vi "AES Encrypt.vi"(0 "Password.In":string, 2 "BitKeyType(256)":u16(ring)=256 items=["AES bit key 128"=128, "AES bit key 192"=192, "AES bit key 256"=256], 7 "PlainText.In":string, 11 "error in":errorcluster, 13 "nonce":u32=123456789) -> (8 "CypheredText out":string, 15 "error out":errorcluster)   [LabVIEW 2020, in "Library Commun.lvlib"]
doc: "AES.Encrypt VI takes string (plain text) and encrypts it with Advanced Encryption Standart (AES) algorithm. \nAES.Encrypt.vi allows reentrant execution.\n-------------------------------------------------------------------------------------------\nThis VI belongs to Server Lab tools at Labicom.net (www.labicom.net) project of remote and virtual laboratories, written by (c) Igor Titov, 2011."
uses:
  Library Commun.lvlib
panel:
  in  "Product information, copyright notice, list of conditions and disclaimer":string="Please visit http://www.labicom.net to learn about remote and virtual laboratories. With it's services and tools you can create remote and/or virtual laboratory and even make money on it.\n \nCopyright (C) 2011 Igor Titov igor.ev.titov@gmail.com\n\nAll rights reserved.\n\nRedistribution and use without modification, are permitted provided that the following conditions are met:\n\n    * Redistributions of source code must retain the above copyright notice, this list of conditions and the following disclaimer.\n    * Redistributions of source code and in binary form may be freely used in all sorts of projects (including commercial ones). It is not obligatory to place copyright notice, this list of conditions and the following disclaimer in your product but you must mention the source (www.labicom.net, Igor Titov) on the web-site of the product.\n    * Neither the name of \"Labicom\", \"labicom.net\", \"Igor Titov\", nor the names of its contributors may be used to endorse or promote products derived from this software without specific prior written permission (except in situations mentioned in the terms and conditions of use of the \"Labicom\").\n\nTHIS SOFTWARE IS PROVIDED BY THE COPYRIGHT HOLDERS AND CONTRIBUTORS \"AS IS\" AND ANY EXPRESS OR IMPLIED WARRANTIES, INCLUDING, BUT NOT LIMITED TO, THE IMPLIED WARRANTIES OF MERCHANTABILITY AND FITNESS FOR A PARTICULAR PURPOSE ARE DISCLAIMED. IN NO EVENT SHALL THE COPYRIGHT OWNER OR CONTRIBUTORS BE LIABLE FOR ANY DIRECT, INDIRECT, INCIDENTAL, SPECIAL, EXEMPLARY, OR CONSEQUENTIAL DAMAGES (INCLUDING, BUT NOT LIMITED TO, PROCUREMENT OF SUBSTITUTE GOODS OR SERVICES; LOSS OF USE, DATA, OR PROFITS; OR BUSINESS INTERRUPTION) HOWEVER CAUSED AND ON ANY THEORY OF LIABILITY, \nWHETHER IN CONTRACT, STRICT LIABILITY, OR TORT (INCLUDING NEGLIGENCE OR OTHERWISE) ARISING IN ANY WAY OUT OF THE USE OF THIS SOFTWARE, EVEN IF ADVISED OF THE POSSIBILITY OF SUCH DAMAGE. "
  in  "Mix Bytes Phases":T1(ring)
  in  "Encryption Phases":T2(ring)
  out "cipherCharStr":string[](array[string])
  out "cipherChar":i32[](array[numeric])
  out "blockLength":i32
  out "cipherCntr":u16[](array[numeric])
  in  "0x100000000":u64=4294967296 format="%.0x"
  out "blockCount":i32
  in  "blockSize":i32=16
  in  "0xff":u16=255 format="%.0x"
  # "Real lab at YOUR home"
  # "Virtual & Remote Laboratories\nwww.labicom.net"
  # "Number of bits used in the key (256 by default).\nThe longer a key, the higher level of protection\nat expence of processor and RAM usage."
  # "Advanced Encryption Standart (AES)\nAES.Encrypt 1.0"
  # "Receives Password in String format (plain text)"
  # "Receives plain text needed to be encrypted"
  # "Encrypted text (with AES)"
  # "o?e?Ae§Oo??)y?B,\no?e?Ae§Oo??)y?B,UoV\"\nQoyµAv"
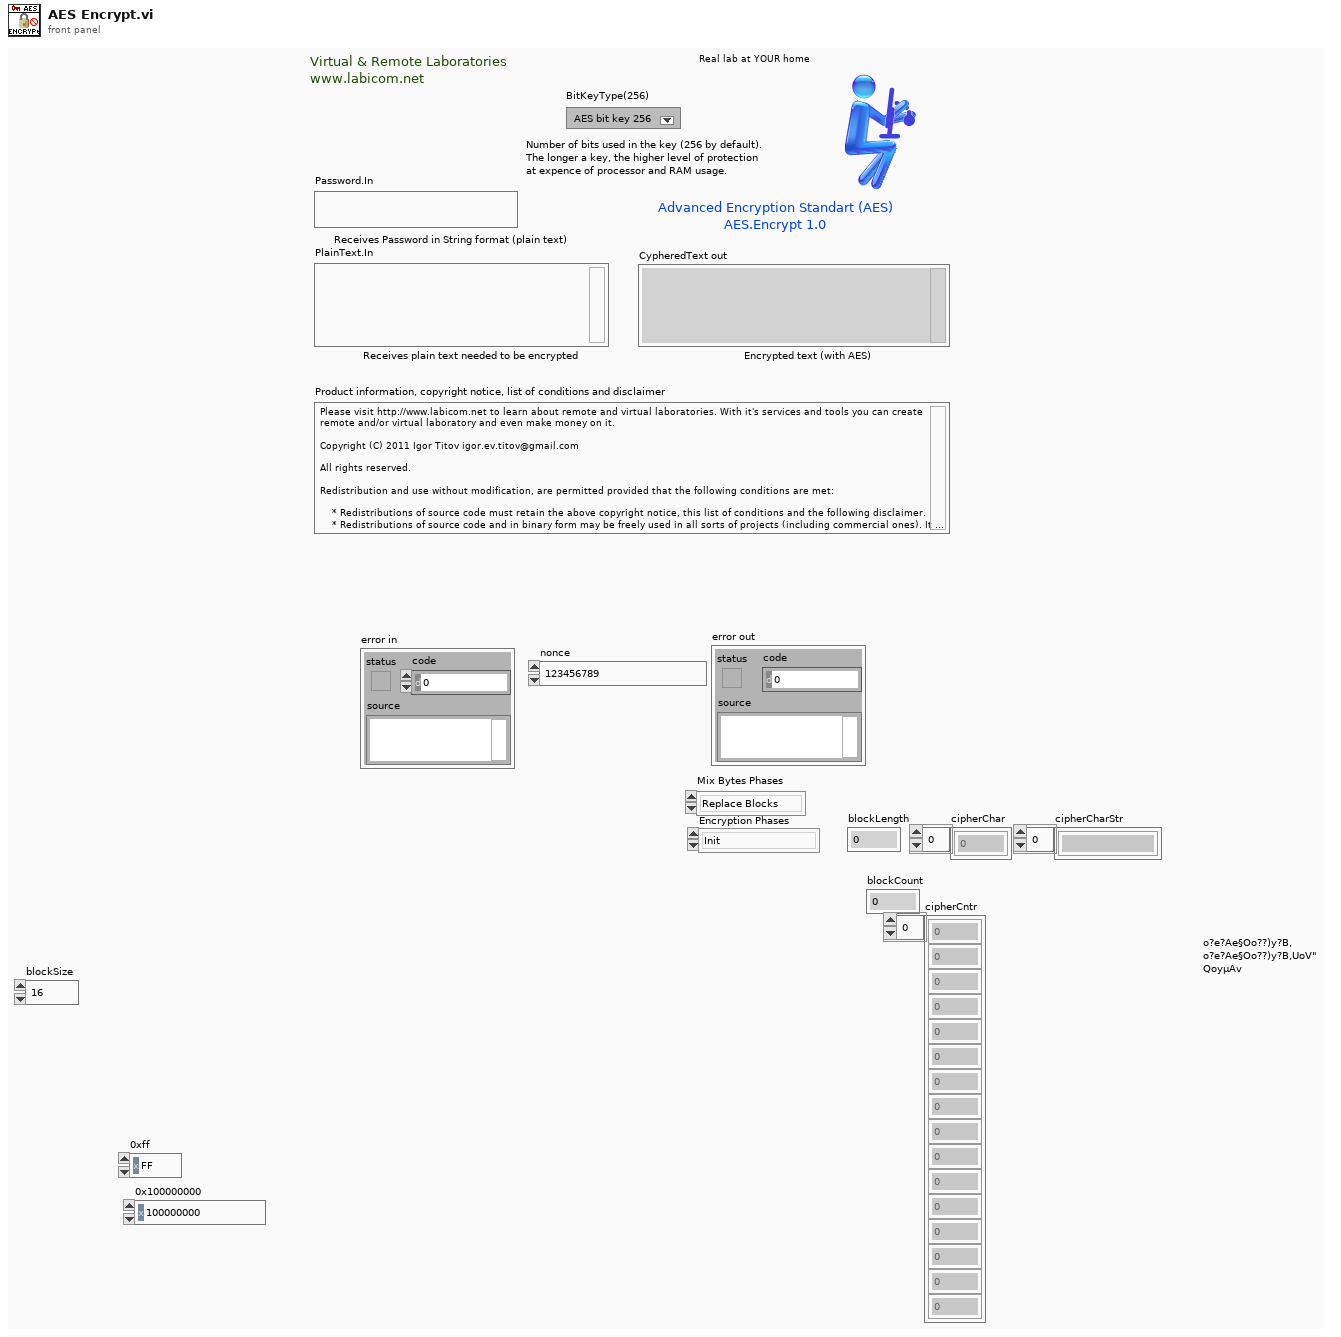
[diagram p1: front panel]
types:
  T1 = enum16{"Replace Blocks", "Cipher Blocks", "Replace ciphered", "Combine parts"}
  T2 = enum16{"Init", "Write pwBytes", "Create Key", "MixBlocks", "ToB64"}
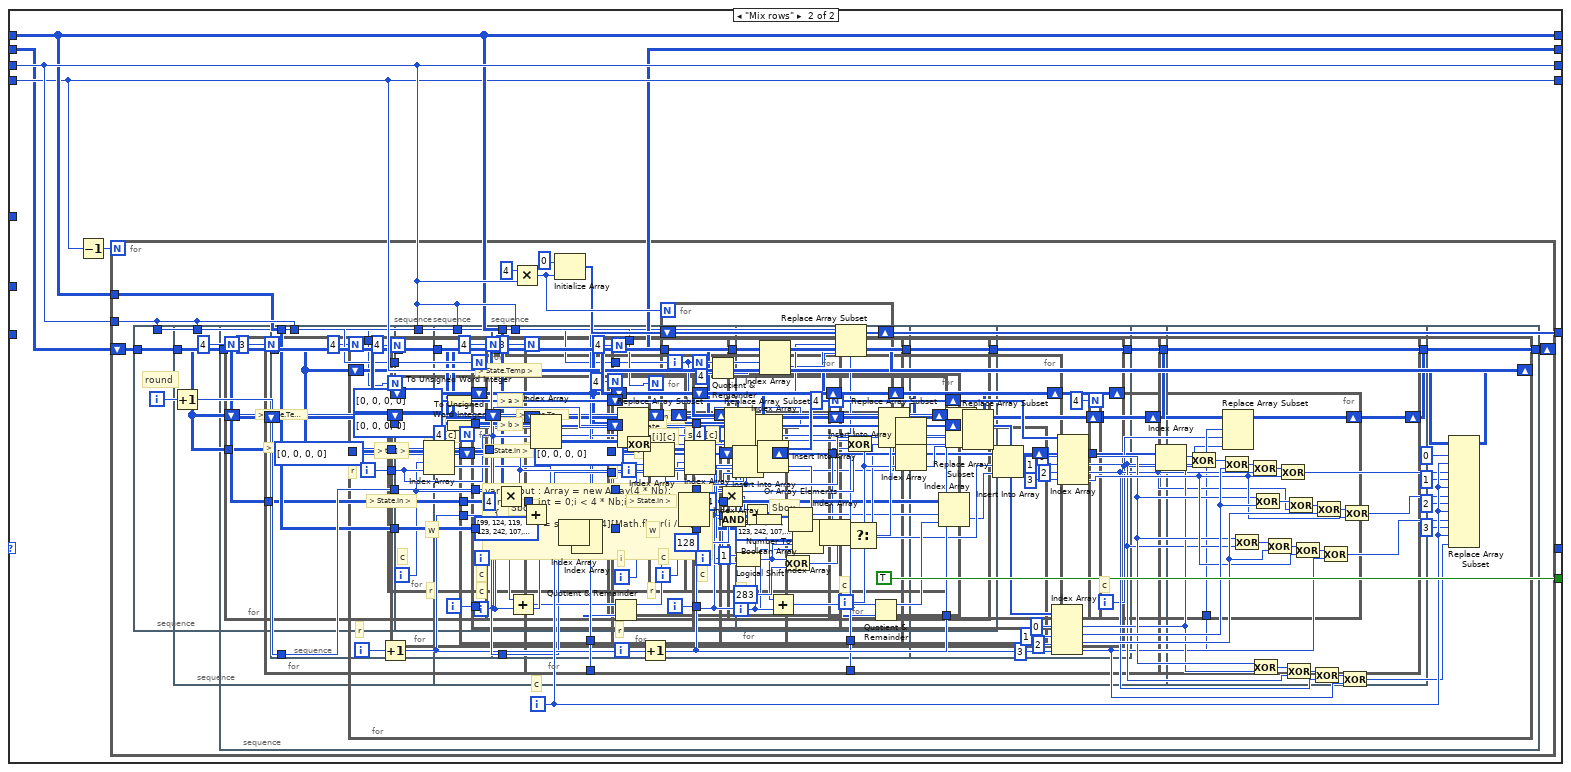
[diagram p4: hidden frame]
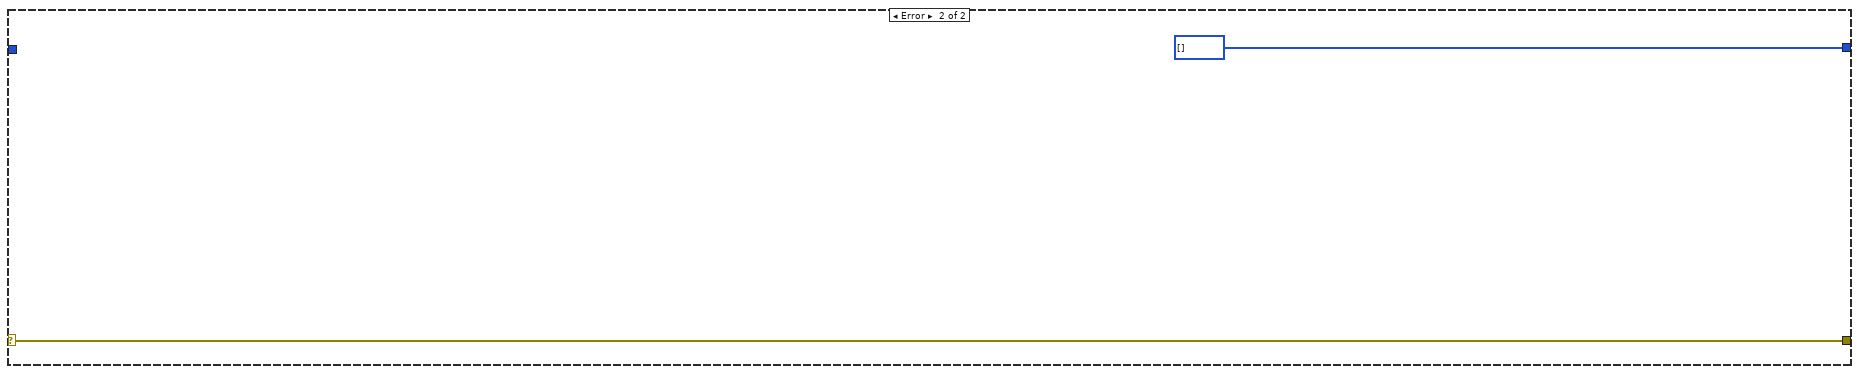
[diagram p5: hidden frame]
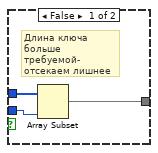
[diagram p6: hidden frame]
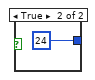
[diagram p7: hidden frame]
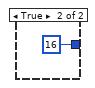
[diagram p8: hidden frame]
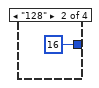
[diagram p9: hidden frame]
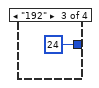
[diagram p10: hidden frame]
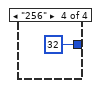
[diagram p11: hidden frame]
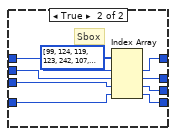
[diagram p12: hidden frame]
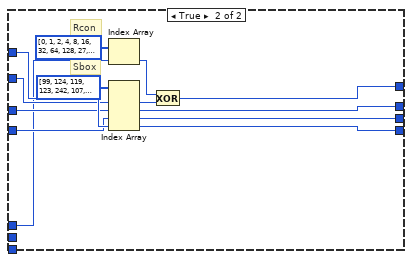
[diagram p13: hidden frame]
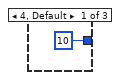
[diagram p14: hidden frame]
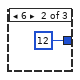
[diagram p15: hidden frame]
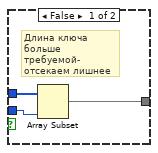
[diagram p16: hidden frame]
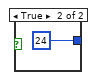
[diagram p17: hidden frame]
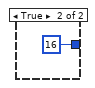
[diagram p18: hidden frame]
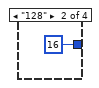
[diagram p19: hidden frame]
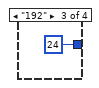
[diagram p20: hidden frame]
diagram:
  n1 = Quotient & Remainder(x="nonce", y=u32 1000) -> (x-y*floor(x/y)=w6:u32, floor(x/y)=w5:u32)
  n2 = case shown="Pas d'erreur" "error in" {
    selector: "error in" -> [w12 w1272]
    tunnel: [w20 w1272] -> w10
    tunnel: "Encryption Phases" -> [w19 _]
    tunnel: w6 -> [w18 _]
    tunnel: w5 -> [w17 _]
    tunnel: "PlainText.In" -> [w16 _]
    tunnel: "Password.In" -> [w15 _]
    tunnel: "BitKeyType(256)" -> [w14 _]
    tunnel: [w13 "" ("Base64 String")] -> w1
    frame No Error {
      n3 = Text to UTF-8(8:w12, 11:w16) -> (0:w20:errorcluster, 3:w21:string)  [unwired: 1 in]
      n4 = while {
        shift-right: [w33] -> _
        shift-left: w19 -> [w49]
        tunnel: w15 -> [w48]
        tunnel: w14 -> [w47]
        shift-right: [w45] -> _
        shift-left: _ -> [w41]
        shift-right: [w44] -> _
        shift-left: _ -> [w40]
        shift-right: [w43] -> _
        shift-left: _ -> [w42]
        shift-right: [w32] -> _
        shift-left: w21 -> [w46]
        shift-right: [w39] -> _
        shift-left: _ -> [w38]
        shift-right: [w37] -> _
        shift-left: _ -> [w36]
        shift-right: [w35] -> _
        shift-left: _ -> [w34]
        shift-right: [w31] -> _
        shift-left: _ -> [w30]
        shift-right: [w29] -> _
        shift-left: _ -> [w28]
        shift-right: [w27] -> _
        shift-left: _ -> [w26]
        tunnel: [w24] -> w13
        tunnel: w18 -> [w23]
        tunnel: w17 -> [w22]
        stop <- w25 stop-if-true
        # "> nonceSec >"
        # "> nonceMs >"
        # "> keySchedule >"
        # "> cipherTxt >"
        # "> ctrTxt >"
        # "> PasswordBytes >"
        # "> blockCount >"
        # "> blockSize >"
        # "> counterBlock >"
        # "> nBytes >"
        # "> PlainText >"
        # "> pwBytes >"
        n5 = case shown="\"Create Key\"" w49 {
          tunnel: w48 -> [w64 _ _ _ _]
          tunnel: w47 -> [w63 _ _ _ _]
          tunnel: w46 -> [w56 w76 w119 w745 w1217]
          tunnel: [w50 w77 w118 w746 w1218] -> w45
          tunnel: [w62 w75 w117 w744 w1216] -> w44
          tunnel: [w61 w84 w116 w743 w1215] -> w43
          tunnel: w42 -> [_ w85 w116 w743 w1215]
          tunnel: w41 -> [_ w77 w118 w746 w1218]
          tunnel: w40 -> [_ w75 w117 w744 w1216]
          tunnel: [w60 w82 w124 w748 w1220] -> w39
          tunnel: w38 -> [_ w83 w124 w748 w1220]
          tunnel: ["blockSize" w81 w120 w747 w1219] -> w37
          tunnel: w36 -> [_ w81 w120 w747 w1219]
          tunnel: [0 w79 w115 w742 w1214] -> w35
          tunnel: w34 -> [_ _ w115 w742 w1214]
          tunnel: [T2."Write pwBytes" ("Encryption Phases") T2."Create Key" ("Encryption Phases") T2."MixBlocks" ("Encryption Phases") T2."ToB64" ("Encryption Phases") T2."Init" ("Encryption Phases")] -> w33
          tunnel: [w56 w76 w119 w745 w1217] -> w32
          tunnel: [w55 w74 w123 w741 w1212] -> w31
          tunnel: w30 -> [_ w74 _ w741 w1212]
          tunnel: [w55 w73 "" w749 w1211] -> w29
          tunnel: w28 -> [_ w73 _ _ w1211]
          tunnel: [u16[] [] ("ExpandedKey") w72 w121 w740 w1213] -> w27
          tunnel: w26 -> [_ w72 _ w740 w1213]
          tunnel: [FALSE FALSE FALSE FALSE TRUE] -> w25
          tunnel: ["" ("Base64 String") _ _ _ w1221] -> w24
          tunnel: w23 -> [_ w71 _ _ _]
          tunnel: w22 -> [_ w70 _ _ _]
          frame "Init", Default {
            w55 = "" ("string")
            # "> counterBlock >"
            # "> pwBytes >"
            # "> nBytes >"
            n6 = Text to UTF-8(11:w64) -> (3:w68:string)  [unwired: 2 in, 1 out]
            n7 = String To Byte Array(string=w68) -> (unsigned byte array=w62:u8[])
            n8 = Divide(x=w63, y=u16 8) -> (x/y=w57:dbl)
            n9 = Initialize Array(u32 0 ("y"), "blockSize") -> (w60:u32[])
            n10 = Initialize Array(u32 0 ("element"), w57) -> (w61:u32[])
            n11 = To Long Integer(number=w57) -> (32bit integer=w50:i32)
          }
          frame "Write pwBytes" {
            # "> blockCount >"
            n12 = String Length(string=w76) -> (length=w87:i32)
            n13 = Divide(x=w87, y=w81) -> (x/y=w88:dbl)
            n14 = Round Toward +Infinity(x=w88) -> (ceil(x): smallest int >= x=w80:dbl)
            n15 = To Long Integer(number=w80) -> (32bit integer=w79:i32)
            "blockCount" <- w79
            n16 = for {
              N: w77 -> [_]
              tunnel: w75 -> [w104] mode=indexing
              shift-right: [w103] -> w84
              shift-left: w85 -> [w102]
              i -> [w106]
              n17 = Not A Number/Path/Refnum?(number/path/refnum=w104) -> (NaN/Path/Refnum?=w108:bool)
              n18 = Select(t=0 ("f"), s=w108, f=w104) -> (s? t:f=w107:i32)
              n19 = Replace Array Subset(array=w102, new element=w107, index=w106) -> (w103:u32[])
            }
            n20 = for {
              N: 4 -> [_]
              shift-right: [w93] -> w82
              shift-left: w83 -> [w92]
              tunnel: w71 -> [w90]
              tunnel: w70 -> [w89]
              i -> [w96]
              w91 = u16 255 ("0xff")
              n21 = Multiply(x=-8, y=w96) -> (x*y=w100:i32)
              n22 = Logical Shift(y=w100, x=w89) -> (x << y=w99:u32)
              n23 = And(x=w99, y=w91) -> (x .and. y?=w98:u32)
              n24 = And(x=w90, y=w91) -> (x .and. y?=w95:u32)
              n25 = Add(x=4, y=w96) -> (x+y=w94:i32)
              n26 = Replace Array Subset(array=w92, new element #1=w98, index #1=w96, new element #2=w95, index #2=w94) -> (w93:u32[])
            }
          }
          frame "Create Key" {
            # "> keySchedule >"
            # "> cipherTxt >"
            # "> ctrTxt >"
            # "> key >"
            n27 = stacked-sequence {
              tunnel: enum16{"128", "192", "256", "auto"}."auto" ("Mode (auto)") -> [w472]
              tunnel: w116 -> [w477]
              tunnel: [w478] -> w126
              frame #0 {
                n28 = Array Size(array=w477) -> (size(s)=w473:i32)
                n29 = case shown="\"auto\", Par défaut" w472 {
                  tunnel: w473 -> [w487 _ _ _]
                  tunnel: [w488 16 24 32] -> w475
                  frame "auto", Default {
                    n30 = Less Or Equal?(x=w487, y=16) -> (x <= y?=w489:bool)
                    n31 = case shown="Faux" w489 {
                      tunnel: [w491 16] -> w488
                      tunnel: w487 -> [w494 _]
                      frame False {
                        n32 = Less Or Equal?(x=w494, y=24) -> (x <= y?=w492:bool)
                        n33 = case shown="Faux" w492 {
                          tunnel: [32 ("y") 24 ("y")] -> w491
                          frame False {
                          }
                          frame True {
                          }
                        }
                      }
                      frame True {
                      }
                    }
                  }
                  frame "128" {
                  }
                  frame "192" {
                  }
                  frame "256" {
                  }
                }
                n34 = Less?(x=w473, y=w475) -> (x < y?=w474:bool)
                n35 = case shown="Vrai" w474 {
                  tunnel: w477 -> [w481 w482]
                  tunnel: w475 -> [w480 w486]
                  tunnel: [w479 w484] -> w476
                  frame False {
                    # "Длина ключа\nбольше требуемой-\nотсекаем лишнее"
                    n36 = Array Subset(array=w481, length=w480) -> (w479:u32[])  [unwired: 1 in]
                  }
                  frame True {
                    # "Длина ключа\nменьше требуемой-\nдополняем нулями"
                    n37 = Initialize Array(u32 0, w486) -> (w485:u32[])
                    n38 = Replace Array Subset(array=w485, new element=w482) -> (w484:u32[])  [unwired: 1 in]
                  }
                }
                n39 = Array Size(array=w476) -> (size(s)=w471:i32)
                n40 = Logical Shift(y=i8 -2, x=w471) -> (x << y=w464:i32)
                n41 = case shown="8" w464 {
                  tunnel: [10 12 14] -> w461
                  frame 4, Default {
                  }
                  frame 6 {
                  }
                  frame 8 {
                  }
                }
                n42 = Increment(x=w461) -> (x+1=w462:i32)
                n43 = Multiply(x=4, y=w462) -> (x*y=w468:i32)
                n44 = Logical Shift(y=i8 2, x=w468) -> (x << y=w467:i32)
                n45 = Initialize Array(u32 0 ("element"), w467) -> (w469:u32[])
                n46 = Replace Array Subset(array=w469, new element=w476) -> (w470:u32[])  [unwired: 1 in]
                n47 = while {
                  tunnel: w468 -> [w553]
                  tunnel: w464 -> [w533]
                  shift-right: [w510] -> w478
                  shift-left: w470 -> [w534]
                  tunnel: w475 -> [w532]
                  i -> [w554]
                  stop <- w552 continue-if-true
                  n48 = Add(x=w533, y=w554) -> (x+y=w536:i32)
                  n49 = Less?(x=w536, y=w553) -> (x < y?=w552:bool)
                  n50 = Quotient & Remainder(x=w536, y=w533) -> (x-y*floor(x/y)=w541:i32, floor(x/y)=w535:i32)
                  n51 = Logical Shift(y=i8 2, x=w536) -> (x << y=w505:i32)
                  n52 = Equal To 0?(x=w541) -> (x = 0?=w542:bool)
                  n53 = Subtract(x=w505, y=4) -> (x-y=w546:i32)
                  n54 = Subtract(x=w505, y=3) -> (x-y=w545:i32)
                  n55 = Subtract(x=w505, y=2) -> (x-y=w544:i32)
                  n56 = Subtract(x=w505, y=1) -> (x-y=w543:i32)
                  n57 = Index Array(array=w534, index #1=w546, index #2=w545, index #3=w544, index #4=w543) -> (element #1=w540:u32, element #2=w539:u32, element #3=w538:u32, element #4=w537:u32)
                  n58 = case shown="Faux" w542 {
                    tunnel: w533 -> [w569 _]
                    tunnel: w541 -> [w567 _]
                    tunnel: w540 -> [w562 w595]
                    tunnel: w539 -> [w561 w594]
                    tunnel: w538 -> [w560 w593]
                    tunnel: w537 -> [w559 w592]
                    tunnel: w535 -> [_ w591]
                    tunnel: [w558 w588] -> w514
                    tunnel: [w557 w587] -> w513
                    tunnel: [w556 w586] -> w512
                    tunnel: [w555 w585] -> w511
                    frame False {
                      n59 = Greater?(x=w569, y=6) -> (0:w565:bool)
                      n60 = Equal?(x=w567, y=4) -> (x = y?=w564:bool)
                      n61 = And(x=w565, y=w564) -> (x .and. y?=w563:bool)
                      n62 = case shown="Faux" w563 {
                        tunnel: w562 -> [w573 w582]
                        tunnel: w561 -> [w572 w581]
                        tunnel: w560 -> [w571 w580]
                        tunnel: w559 -> [w570 w579]
                        tunnel: [w573 w578] -> w558
                        tunnel: [w572 w577] -> w557
                        tunnel: [w571 w576] -> w556
                        tunnel: [w570 w575] -> w555
                        frame False {
                        }
                        frame True {
                          # "Sbox"
                          n63 = Index Array(array=u32[] [99, 124, 119, 123, 242, 107, 111, 197, 48, 1, 103, 43, 254, 215, 171, 118, 202, 130, 201, 125, 250, 89, 71, 240, 173, 212, 162, 175, 156, 164, 114, 192, 183, 253, 147, 38, 54, 63, 247, 204, 52, 165, 229, 241, 113, 216, 49, 21, 4, 199, 35, 195, 24, 150, 5, 154, 7, 18, 128, 226, 235, 39, 178, 117, 9, 131, 44, 26, 27, 110, 90, 160, 82, 59, 214, 179, 41, 227, 47, 132, 83, 209, 0, 237, 32, 252, 177, 91, 106, 203, 190, 57, 74, 76, 88, 207, 208, 239, 170, 251, 67, 77, 51, 133, 69, 249, 2, 127, 80, 60, 159, 168, 81, 163, 64, 143, 146, 157, 56, 245, 188, 182, 218, 33, 16, 255, 243, 210, 205, 12, 19, 236, 95, 151, 68, 23, 196, 167, 126, 61, 100, 93, 25, 115, 96, 129, 79, 220, 34, 42, 144, 136, 70, 238, 184, 20, 222, 94, 11, 219, 224, 50, 58, 10, 73, 6, 36, 92, 194, 211, 172, 98, 145, 149, 228, 121, 231, 200, 55, 109, 141, 213, 78, 169, 108, 86, 244, 234, 101, 122, 174, 8, 186, 120, 37, 46, 28, 166, 180, 198, 232, 221, 116, 31, 75, 189, 139, 138, 112, 62, 181, 102, 72, 3, 246, 14, 97, 53, 87, 185, 134, 193, 29, 158, 225, 248, 152, 17, 105, 217, 142, 148, 155, 30, 135, 233, 206, 85, 40, 223, 140, 161, 137, 13, 191, 230, 66, 104, 65, 153, 45, 15, 176, 84, 187, 22] ("Sbox"), index #1=w582, index #2=w581, index #3=w580, index #4=w579) -> (element #1=w578:u32, element #2=w577:u32, element #3=w576:u32, element #4=w575:u32)
                        }
                      }
                    }
                    frame True {
                      # "Sbox"
                      # "Rcon"
                      n64 = Index Array(array=u32[] [0, 1, 2, 4, 8, 16, 32, 64, 128, 27, 54] ("Rcon"), index=w591) -> (element=w590:u32)
                      n65 = Index Array(array=u32[] [99, 124, 119, 123, 242, 107, 111, 197, 48, 1, 103, 43, 254, 215, 171, 118, 202, 130, 201, 125, 250, 89, 71, 240, 173, 212, 162, 175, 156, 164, 114, 192, 183, 253, 147, 38, 54, 63, 247, 204, 52, 165, 229, 241, 113, 216, 49, 21, 4, 199, 35, 195, 24, 150, 5, 154, 7, 18, 128, 226, 235, 39, 178, 117, 9, 131, 44, 26, 27, 110, 90, 160, 82, 59, 214, 179, 41, 227, 47, 132, 83, 209, 0, 237, 32, 252, 177, 91, 106, 203, 190, 57, 74, 76, 88, 207, 208, 239, 170, 251, 67, 77, 51, 133, 69, 249, 2, 127, 80, 60, 159, 168, 81, 163, 64, 143, 146, 157, 56, 245, 188, 182, 218, 33, 16, 255, 243, 210, 205, 12, 19, 236, 95, 151, 68, 23, 196, 167, 126, 61, 100, 93, 25, 115, 96, 129, 79, 220, 34, 42, 144, 136, 70, 238, 184, 20, 222, 94, 11, 219, 224, 50, 58, 10, 73, 6, 36, 92, 194, 211, 172, 98, 145, 149, 228, 121, 231, 200, 55, 109, 141, 213, 78, 169, 108, 86, 244, 234, 101, 122, 174, 8, 186, 120, 37, 46, 28, 166, 180, 198, 232, 221, 116, 31, 75, 189, 139, 138, 112, 62, 181, 102, 72, 3, 246, 14, 97, 53, 87, 185, 134, 193, 29, 158, 225, 248, 152, 17, 105, 217, 142, 148, 155, 30, 135, 233, 206, 85, 40, 223, 140, 161, 137, 13, 191, 230, 66, 104, 65, 153, 45, 15, 176, 84, 187, 22] ("Sbox"), index #1=w594, index #2=w593, index #3=w592, index #4=w595) -> (element #1=w589:u32, element #2=w587:u32, element #3=w586:u32, element #4=w585:u32)
                      n66 = Exclusive Or(1:w589, 2:w590) -> (0:w588:u32)
                    }
                  }
                  n67 = Subtract(x=w505, y=w532) -> (x-y=w531:i32)
                  n68 = Add(x=w531, y=0) -> (x+y=w526:i32)
                  n69 = Add(x=w531, y=1) -> (x+y=w525:i32)
                  n70 = Add(x=w531, y=2) -> (x+y=w524:i32)
                  n71 = Add(x=w531, y=3) -> (x+y=w523:i32)
                  n72 = Index Array(array=w534, index #1=w526, index #2=w525, index #3=w524, index #4=w523) -> (element #1=w522:u32, element #2=w521:u32, element #3=w520:u32, element #4=w519:u32)
                  n73 = Exclusive Or(1:w514, 2:w522) -> (0:w518:u32)
                  n74 = Exclusive Or(1:w513, 2:w521) -> (0:w517:u32)
                  n75 = Exclusive Or(1:w512, 2:w520) -> (0:w516:u32)
                  n76 = Exclusive Or(1:w511, 2:w519) -> (0:w515:u32)
                  n77 = Add(x=w505, y=0) -> (x+y=w504:i32)
                  n78 = Add(x=w505, y=1) -> (x+y=w503:i32)
                  n79 = Add(x=w505, y=2) -> (x+y=w502:i32)
                  n80 = Add(x=w505, y=3) -> (x+y=w501:i32)
                  n81 = Replace Array Subset(array=w534, new element #1=w518, index #1=w504, new element #2=w517, index #2=w503, new element #3=w516, index #3=w502, new element #4=w515, index #4=w501) -> (w510:u32[])
                }
              }
            }
            n82 = Split 1D Array(array=w124, index=8) -> (first subarray=w135:u32[])  [unwired: 1 out]
            n83 = Subtract(x=w118, y=u8 16) -> (x-y=w131:i32)
            n84 = stacked-sequence {
              tunnel: w116 -> [w139]
              tunnel: [w140] -> w127
              tunnel: w126 -> [w138]
              tunnel: errorcluster {"status"=FALSE, "code"=0, "source"=""} ("error in") -> [w136]
              tunnel: [w137] -> _
              frame #0 {
                n85 = case shown="Pas d'erreur" w136 {
                  selector: w136 -> [_ w459]
                  tunnel: [_ w459] -> w137
                  tunnel: w138 -> [w145 _]
                  tunnel: w139 -> [w144 _]
                  tunnel: [w143 u16[] []] -> w140
                  tunnel: 4 ("Nb") -> [w142 _]
                  frame No Error {
                    n86 = while {
                      shift-right: [w149] -> _
                      shift-left: enum16{"Init", "Mix rows"}."Init" ("Cipher Phases") -> [w161]
                      tunnel: w145 -> [w160]
                      tunnel: w144 -> [w159]
                      shift-right: [w158] -> _
                      shift-left: _ -> [w157]
                      shift-right: [w156] -> _
                      shift-left: _ -> [w155]
                      shift-right: [w154] -> _
                      shift-left: _ -> [w153]
                      shift-right: [w152] -> _
                      shift-left: _ -> [w151]
                      tunnel: [w150] -> w143
                      tunnel: w142 -> [w147]
                      stop <- w148 stop-if-true
                      # "> Nr >"
                      # "> Nb >"
                      # "> State >"
                      # "> ExpandedKez(w)(2D) >"
                      n87 = case shown="\"Init\", Par défaut" w161 {
                        tunnel: w160 -> [w174 _]
                        tunnel: w159 -> [w172 _]
                        tunnel: [w169 w222] -> w158
                        tunnel: w157 -> [_ w222]
                        tunnel: [w168 w215] -> w156
                        tunnel: w155 -> [_ w216]
                        tunnel: [w162 w223] -> w154
                        tunnel: w153 -> [_ w223]
                        tunnel: [w166 w221] -> w152
                        tunnel: w151 -> [_ w221]
                        tunnel: [_ w218] -> w150
                        tunnel: [enum16{"Init", "Mix rows"}."Mix rows" ("Cipher Phases") _] -> w149
                        tunnel: [FALSE TRUE] -> w148
                        tunnel: w147 -> [w162 _]
                        frame "Init", Default {
                          # "> Nb >"
                          # "> ExpandedKey(w)(2D) >"
                          # "> Nr >"
                          n88 = Reshape Array(w174, 60 ("dimension size"), 4 ("dimension size")) -> (w169:u32[][])
                          n89 = for {
                            N: 16 -> [_]
                            tunnel: w172 -> [w209]
                            shift-right: [w207] -> w170
                            shift-left: u16[][] [[0, 0, 0, 0], [0, 0, 0, 0], [0, 0, 0, 0], [0, 0, 0, 0]] ("State.Out") -> [w208]
                            i -> [w214]
                            n90 = Quotient & Remainder(x=w214, y=4) -> (x-y*floor(x/y)=w211:i32, floor(x/y)=w210:i32)
                            n91 = Index Array(array=w209, index=w214) -> (element=w212:u32)
                            n92 = Replace Array Subset(array=w208, new element=w212, index (row)=w211, index (col)=w210) -> (w207:u16[][])
                          }
                          n93 = Array Size(array=w169) -> (size(s)=w175:i32[])
                          n94 = Index Array(array=w175, index=0) -> (element=w178:i32)
                          n95 = Divide(x=w178, y=w162) -> (x/y=w177:dbl)
                          n96 = Decrement(x=w177) -> (x-1=w167:dbl)
                          n97 = To Long Integer(number=w167) -> (32bit integer=w166:i32)
                          n98 = stacked-sequence {
                            tunnel: w169 -> [w181]
                            tunnel: w162 -> [w183]
                            tunnel: w170 -> [w185]
                            tunnel: [w186] -> w168
                            tunnel: 0 ("rnd (0)") -> [w184]
                            frame #0 {
                              n99 = for {
                                N: 4 -> [_]
                                tunnel: w185 -> [w192]
                                tunnel: w181 -> [w191]
                                tunnel: w183 -> [w190]
                                tunnel: w184 -> [w189]
                                shift-right: [w187] -> w186
                                shift-left: w185 -> [w188]
                                i -> [w193]
                                # "w"
                                # "state"
                                # "r"
                                n100 = for {
                                N: w190 -> [_]
                                tunnel: w193 -> [w198]
                                tunnel: w192 -> [w201]
                                tunnel: w191 -> [w206]
                                tunnel: w189 -> [w205]
                                shift-right: [w194] -> w187
                                shift-left: w188 -> [w195]
                                i -> [w197]
                                # "c"
                                n101 = Multiply(x=w205, y=4) -> (x*y=w203:i32)
                                n102 = Add(x=w203, y=w197) -> (x+y=w202:i32)
                                n103 = Index Array(array=w201, index (row)=w198, index (col)=w197) -> (element=w200:u16)
                                n104 = Index Array(array=w206, index (row)=w202, index (col)=w198) -> (element=w199:u32)
                                n105 = Exclusive Or(1:w199, 2:w200) -> (0:w196:u32)
                                n106 = Replace Array Subset(array=w195, new element=w196, index (row)=w198, index (col)=w197) -> (w194:u16[][])
                                }
                              }
                            }
                          }
                        }
                        frame "Mix rows" {
                          # "var output : Array = new Array(4 * Nb); \n\tfor (var i : int = 0;i < 4 * Nb;i++)\n   {\n    output[i] = state[i % 4][Math.floor(i / 4)];\n\t\t\t}"
                          n107 = Decrement(x=w221) -> (x-1=w229:i32)
                          n108 = for {
                            N: w229 -> [_]
                            shift-right: [w312] -> w224
                            shift-left: w216 -> [w313]
                            tunnel: w223 -> [w311]
                            tunnel: w222 -> [w310]
                            i -> [w315]
                            # "round"
                            n109 = stacked-sequence {
                              tunnel: w311 -> [w319]
                              tunnel: w313 -> [w321]
                              tunnel: [w322] -> w318
                              frame #0 {
                                n110 = for {
                                N: 4 -> [_]
                                tunnel: w321 -> [w326]
                                shift-right: [w323] -> w322
                                shift-left: w321 -> [w325]
                                tunnel: w319 -> [w324]
                                i -> [w327]
                                # "> State.In >"
                                # "> State.Temp >"
                                # "r"
                                n111 = for {
                                N: w324 -> [_]
                                tunnel: w326 -> [w335]
                                tunnel: w327 -> [w332]
                                shift-right: [w328] -> w323
                                shift-left: w325 -> [w329]
                                i -> [w331]
                                # "Sbox"
                                # "s[r][c]"
                                # "c"
                                n112 = Index Array(array=w335, index (row)=w331, index (col)=w332) -> (element=w334:u16)
                                n113 = Index Array(array=u16[] [99, 124, 119, 123, 242, 107, 111, 197, 48, 1, 103, 43, 254, 215, 171, 118, 202, 130, 201, 125, 250, 89, 71, 240, 173, 212, 162, 175, 156, 164, 114, 192, 183, 253, 147, 38, 54, 63, 247, 204, 52, 165, 229, 241, 113, 216, 49, 21, 4, 199, 35, 195, 24, 150, 5, 154, 7, 18, 128, 226, 235, 39, 178, 117, 9, 131, 44, 26, 27, 110, 90, 160, 82, 59, 214, 179, 41, 227, 47, 132, 83, 209, 0, 237, 32, 252, 177, 91, 106, 203, 190, 57, 74, 76, 88, 207, 208, 239, 170, 251, 67, 77, 51, 133, 69, 249, 2, 127, 80, 60, 159, 168, 81, 163, 64, 143, 146, 157, 56, 245, 188, 182, 218, 33, 16, 255, 243, 210, 205, 12, 19, 236, 95, 151, 68, 23, 196, 167, 126, 61, 100, 93, 25, 115, 96, 129, 79, 220, 34, 42, 144, 136, 70, 238, 184, 20, 222, 94, 11, 219, 224, 50, 58, 10, 73, 6, 36, 92, 194, 211, 172, 98, 145, 149, 228, 121, 231, 200, 55, 109, 141, 213, 78, 169, 108, 86, 244, 234, 101, 122, 174, 8, 186, 120, 37, 46, 28, 166, 180, 198, 232, 221, 116, 31, 75, 189, 139, 138, 112, 62, 181, 102, 72, 3, 246, 14, 97, 53, 87, 185, 134, 193, 29, 158, 225, 248, 152, 17, 105, 217, 142, 148, 155, 30, 135, 233, 206, 85, 40, 223, 140, 161, 137, 13, 191, 230, 66, 104, 65, 153, 45, 15, 176, 84, 187, 22] ("Sbox"), index=w334) -> (element=w333:u16)
                                n114 = Replace Array Subset(array=w329, new element=w333, index (row)=w331, index (col)=w332) -> (w328:u16[][])
                                }
                                }
                              }
                            }
                            n115 = Increment(x=w315) -> (x+1=w314:i32)
                            n116 = stacked-sequence {
                              tunnel: w311 -> [w336]
                              tunnel: w318 -> [w338]
                              tunnel: [w339] -> w317
                              frame #0 {
                                n117 = for {
                                N: 3 -> [_]
                                tunnel: w338 -> [w349]
                                shift-right: [w345] -> w339
                                shift-left: w338 -> [w346]
                                tunnel: w336 -> [w340]
                                i -> [w348]
                                # "> t[c] >"
                                # "> State.In >"
                                # "> State.Temp >"
                                # "r"
                                n118 = Increment(x=w348) -> (x+1=w347:i32)
                                n119 = for {
                                N: 4 -> [_]
                                tunnel: w349 -> [w364]
                                tunnel: w347 -> [w360]
                                shift-right: [w356] -> w343
                                shift-left: i32[] [0, 0, 0, 0] ("t[c]") -> [w357]
                                tunnel: w340 -> [w362]
                                i -> [w359]
                                # "c"
                                n120 = Add(x=w360, y=w359) -> (x+y=w363:i32)
                                n121 = Quotient & Remainder(x=w363, y=w362) -> (x-y*floor(x/y)=w361:i32)  [unwired: 1 out]
                                n122 = Index Array(array=w364, index (row)=w360, index (col)=w361) -> (element=w358:u16)
                                n123 = Insert Into Array(array=w357, index=w359, new element=w358) -> (w356:i32[])
                                }
                                n124 = for {
                                N: 4 -> [_]
                                tunnel: w347 -> [w355]
                                shift-right: [w351] -> w345
                                shift-left: w346 -> [w352]
                                tunnel: w343 -> [w350]
                                i -> [w354]
                                # "c"
                                n125 = Index Array(array=w350, index=w354) -> (element=w353:i32)
                                n126 = Replace Array Subset(array=w352, new element=w353, index (row)=w355, index (col)=w354) -> (w351:u16[][])
                                }
                                }
                              }
                            }
                            n127 = stacked-sequence {
                              tunnel: w317 -> [w366]
                              tunnel: [w367] -> w316
                              frame #0 {
                                n128 = for {
                                N: 4 -> [_]
                                shift-right: [w411] -> w367
                                shift-left: w366 -> [w412]
                                tunnel: w366 -> [w413]
                                i -> [w414]
                                # "> b >"
                                # "> a >"
                                # "> State.In >"
                                # "> State.Temp >"
                                # "c"
                                n129 = To Unsigned Word Integer(number=i32[] [0, 0, 0, 0] ("t[c]")) -> (unsigned 16bit integer=w408:u16[])
                                n130 = To Unsigned Word Integer(number=i32[] [0, 0, 0, 0] ("t[c]")) -> (unsigned 16bit integer=w407:u16[])
                                n131 = for {
                                N: 4 -> [_]
                                tunnel: w413 -> [w431]
                                tunnel: w414 -> [w430]
                                shift-right: [w417] -> w406
                                shift-left: w408 -> [w418]
                                shift-right: [w415] -> w405
                                shift-left: w407 -> [w416]
                                i -> [w429]
                                # "s[i][c]"
                                # "i"
                                n132 = Index Array(array=w431, index (row)=w429, index (col)=w430) -> (element=w423:u16)
                                n133 = And(x=w423, y=u16 128 ("0x80")) -> (x .and. y?=w426:u16)
                                n134 = Logical Shift(y=i8 1, x=w423) -> (x << y=w420:u16)
                                n135 = Number To Boolean Array(number=w426) -> (Boolean array=w425:bool[])
                                n136 = Insert Into Array(array=w418, index=w429, new element=w423) -> (w417:u16[])
                                n137 = Exclusive Or(1:u16 283 ("0x011b"), 2:w420) -> (0:w421:u16)
                                n138 = Or Array Elements(Boolean array=w425) -> (logical OR=w424:bool)
                                n139 = Select(t=w421, s=w424, f=w420) -> (s? t:f=w428:u16)
                                n140 = Insert Into Array(array=w416, index=w429, new element=w428) -> (w415:u16[])
                                }
                                n141 = Index Array(array=w405, index #1=0 ("index"), index #2=1 ("index"), index #3=2 ("index"), index #4=3 ("index")) -> (element #1=w376:u16, element #2=w388:u16, element #3=w383:u16, element #4=w373:u16)
                                n142 = Index Array(array=w406, index #1=0 ("index"), index #2=1 ("index"), index #3=2 ("index"), index #4=3 ("index")) -> (element #1=w377:u16, element #2=w375:u16, element #3=w374:u16, element #4=w382:u16)
                                n143 = Exclusive Or(1:w375, 2:w376) -> (0:w395:u16)
                                n144 = Exclusive Or(1:w388, 2:w395) -> (0:w394:u16)
                                n145 = Exclusive Or(1:w375, 2:w377) -> (0:w386:u16)
                                n146 = Exclusive Or(1:w374, 2:w394) -> (0:w393:u16)
                                n147 = Exclusive Or(1:w376, 2:w377) -> (0:w380:u16)
                                n148 = Exclusive Or(1:w388, 2:w377) -> (0:w391:u16)
                                n149 = Exclusive Or(1:w383, 2:w386) -> (0:w385:u16)
                                n150 = Exclusive Or(1:w382, 2:w393) -> (0:w392:u16)
                                n151 = Exclusive Or(1:w375, 2:w380) -> (0:w379:u16)
                                n152 = Exclusive Or(1:w374, 2:w391) -> (0:w390:u16)
                                n153 = Exclusive Or(1:w382, 2:w385) -> (0:w384:u16)
                                n154 = Exclusive Or(1:w374, 2:w379) -> (0:w378:u16)
                                n155 = Exclusive Or(1:w383, 2:w390) -> (0:w389:u16)
                                n156 = Exclusive Or(1:w373, 2:w384) -> (0:w381:u16)
                                n157 = Exclusive Or(1:w373, 2:w378) -> (0:w372:u16)
                                n158 = Exclusive Or(1:w382, 2:w389) -> (0:w387:u16)
                                n159 = Replace Array Subset(array=w412, new element #1=w392, index (row) #1=0 ("disabled index (col)"), index (col) #1=w414, new element #2=w387, index (row) #2=1 ("disabled index (col)"), index (col) #2=w414, new element #3=w381, index (row) #3=2 ("disabled index (col)"), index (col) #3=w414, new element #4=w372, index (row) #4=3 ("disabled index (col)"), index (col) #4=w414) -> (w411:u16[][])
                                }
                              }
                            }
                            n160 = stacked-sequence {
                              tunnel: w310 -> [w432]
                              tunnel: w311 -> [w434]
                              tunnel: w316 -> [w436]
                              tunnel: [w437] -> w312
                              tunnel: w314 -> [w435]
                              frame #0 {
                                n161 = for {
                                N: 4 -> [_]
                                tunnel: w436 -> [w443]
                                tunnel: w432 -> [w442]
                                tunnel: w434 -> [w441]
                                tunnel: w435 -> [w440]
                                shift-right: [w438] -> w437
                                shift-left: w436 -> [w439]
                                i -> [w444]
                                # "w"
                                # "state"
                                # "r"
                                n162 = for {
                                N: w441 -> [_]
                                tunnel: w444 -> [w449]
                                tunnel: w443 -> [w452]
                                tunnel: w442 -> [w457]
                                tunnel: w440 -> [w456]
                                shift-right: [w445] -> w438
                                shift-left: w439 -> [w446]
                                i -> [w448]
                                # "c"
                                n163 = Multiply(x=w456, y=4) -> (x*y=w454:i32)
                                n164 = Add(x=w454, y=w448) -> (x+y=w453:i32)
                                n165 = Index Array(array=w452, index (row)=w449, index (col)=w448) -> (element=w451:u16)
                                n166 = Index Array(array=w457, index (row)=w453, index (col)=w449) -> (element=w450:u32)
                                n167 = Exclusive Or(1:w450, 2:w451) -> (0:w447:u32)
                                n168 = Replace Array Subset(array=w446, new element=w447, index (row)=w449, index (col)=w448) -> (w445:u16[][])
                                }
                                }
                              }
                            }
                          }
                          n169 = stacked-sequence {
                            tunnel: w223 -> [w285]
                            tunnel: w224 -> [w287]
                            tunnel: [w288] -> w228
                            frame #0 {
                              n170 = for {
                                N: 4 -> [_]
                                tunnel: w287 -> [w292]
                                shift-right: [w289] -> w288
                                shift-left: w287 -> [w291]
                                tunnel: w285 -> [w290]
                                i -> [w293]
                                # "> State.In >"
                                # "> State.Temp >"
                                # "r"
                                n171 = for {
                                N: w290 -> [_]
                                tunnel: w292 -> [w301]
                                tunnel: w293 -> [w298]
                                shift-right: [w294] -> w289
                                shift-left: w291 -> [w295]
                                i -> [w297]
                                # "Sbox"
                                # "s[r][c]"
                                # "c"
                                n172 = Index Array(array=w301, index (row)=w297, index (col)=w298) -> (element=w300:u16)
                                n173 = Index Array(array=u16[] [99, 124, 119, 123, 242, 107, 111, 197, 48, 1, 103, 43, 254, 215, 171, 118, 202, 130, 201, 125, 250, 89, 71, 240, 173, 212, 162, 175, 156, 164, 114, 192, 183, 253, 147, 38, 54, 63, 247, 204, 52, 165, 229, 241, 113, 216, 49, 21, 4, 199, 35, 195, 24, 150, 5, 154, 7, 18, 128, 226, 235, 39, 178, 117, 9, 131, 44, 26, 27, 110, 90, 160, 82, 59, 214, 179, 41, 227, 47, 132, 83, 209, 0, 237, 32, 252, 177, 91, 106, 203, 190, 57, 74, 76, 88, 207, 208, 239, 170, 251, 67, 77, 51, 133, 69, 249, 2, 127, 80, 60, 159, 168, 81, 163, 64, 143, 146, 157, 56, 245, 188, 182, 218, 33, 16, 255, 243, 210, 205, 12, 19, 236, 95, 151, 68, 23, 196, 167, 126, 61, 100, 93, 25, 115, 96, 129, 79, 220, 34, 42, 144, 136, 70, 238, 184, 20, 222, 94, 11, 219, 224, 50, 58, 10, 73, 6, 36, 92, 194, 211, 172, 98, 145, 149, 228, 121, 231, 200, 55, 109, 141, 213, 78, 169, 108, 86, 244, 234, 101, 122, 174, 8, 186, 120, 37, 46, 28, 166, 180, 198, 232, 221, 116, 31, 75, 189, 139, 138, 112, 62, 181, 102, 72, 3, 246, 14, 97, 53, 87, 185, 134, 193, 29, 158, 225, 248, 152, 17, 105, 217, 142, 148, 155, 30, 135, 233, 206, 85, 40, 223, 140, 161, 137, 13, 191, 230, 66, 104, 65, 153, 45, 15, 176, 84, 187, 22] ("Sbox"), index=w300) -> (element=w299:u16)
                                n174 = Replace Array Subset(array=w295, new element=w299, index (row)=w297, index (col)=w298) -> (w294:u16[][])
                                }
                              }
                            }
                          }
                          n175 = stacked-sequence {
                            tunnel: w223 -> [w256]
                            tunnel: w228 -> [w258]
                            tunnel: [w259] -> w227
                            frame #0 {
                              n176 = for {
                                N: 3 -> [_]
                                tunnel: w258 -> [w269]
                                shift-right: [w265] -> w259
                                shift-left: w258 -> [w266]
                                tunnel: w256 -> [w260]
                                i -> [w268]
                                # "> t[c] >"
                                # "> State.In >"
                                # "> State.Temp >"
                                # "r"
                                n177 = Increment(x=w268) -> (x+1=w267:i32)
                                n178 = for {
                                N: 4 -> [_]
                                tunnel: w269 -> [w284]
                                tunnel: w267 -> [w280]
                                shift-right: [w276] -> w263
                                shift-left: i32[] [0, 0, 0, 0] ("t[c]") -> [w277]
                                tunnel: w260 -> [w282]
                                i -> [w279]
                                # "c"
                                n179 = Add(x=w280, y=w279) -> (x+y=w283:i32)
                                n180 = Quotient & Remainder(x=w283, y=w282) -> (x-y*floor(x/y)=w281:i32)  [unwired: 1 out]
                                n181 = Index Array(array=w284, index (row)=w280, index (col)=w281) -> (element=w278:u16)
                                n182 = Insert Into Array(array=w277, index=w279, new element=w278) -> (w276:i32[])
                                }
                                n183 = for {
                                N: 4 -> [_]
                                tunnel: w267 -> [w275]
                                shift-right: [w271] -> w265
                                shift-left: w266 -> [w272]
                                tunnel: w263 -> [w270]
                                i -> [w274]
                                # "c"
                                n184 = Index Array(array=w270, index=w274) -> (element=w273:i32)
                                n185 = Replace Array Subset(array=w272, new element=w273, index (row)=w275, index (col)=w274) -> (w271:u16[][])
                                }
                              }
                            }
                          }
                          n186 = stacked-sequence {
                            tunnel: w222 -> [w230]
                            tunnel: w223 -> [w232]
                            tunnel: w227 -> [w234]
                            tunnel: [w235] -> w215
                            tunnel: w221 -> [w233]
                            frame #0 {
                              n187 = for {
                                N: 4 -> [_]
                                tunnel: w234 -> [w241]
                                tunnel: w230 -> [w240]
                                tunnel: w232 -> [w239]
                                tunnel: w233 -> [w238]
                                shift-right: [w236] -> w235
                                shift-left: w234 -> [w237]
                                i -> [w242]
                                # "w"
                                # "state"
                                # "r"
                                n188 = for {
                                N: w239 -> [_]
                                tunnel: w242 -> [w247]
                                tunnel: w241 -> [w250]
                                tunnel: w240 -> [w255]
                                tunnel: w238 -> [w254]
                                shift-right: [w243] -> w236
                                shift-left: w237 -> [w244]
                                i -> [w246]
                                # "c"
                                n189 = Multiply(x=w254, y=4) -> (x*y=w252:i32)
                                n190 = Add(x=w252, y=w246) -> (x+y=w251:i32)
                                n191 = Index Array(array=w250, index (row)=w247, index (col)=w246) -> (element=w249:u16)
                                n192 = Index Array(array=w255, index (row)=w251, index (col)=w247) -> (element=w248:u32)
                                n193 = Exclusive Or(1:w248, 2:w249) -> (0:w245:u32)
                                n194 = Replace Array Subset(array=w244, new element=w245, index (row)=w247, index (col)=w246) -> (w243:u16[][])
                                }
                              }
                            }
                          }
                          n195 = Multiply(x=4, y=w223) -> (x*y=w220:i32)
                          n196 = Initialize Array(u16 0 ("x"), w220) -> (w219:u16[])
                          n197 = for {
                            N: w220 -> [_]
                            shift-right: [w302] -> w218
                            shift-left: w219 -> [w303]
                            tunnel: w215 -> [w304]
                            i -> [w306]
                            n198 = Quotient & Remainder(x=w306, y=4) -> (x-y*floor(x/y)=w308:i32, floor(x/y)=w307:i32)
                            n199 = Index Array(array=w304, index (row)=w308, index (col)=w307) -> (element=w305:u16)
                            n200 = Replace Array Subset(array=w303, new element=w305, index=w306) -> (w302:u16[])
                          }
                        }
                      }
                    }
                  }
                  frame Error {
                  }
                }
              }
            }
            n201 = Byte Array To String(unsigned byte array=w135) -> (string=w123:string)
            n202 = Byte Array To String(unsigned byte array=w127) -> (string=w128:string)
            n203 = String Subset(string=w128, offset (0)=0, length (rest)=w131) -> (substring=w132:string)
            n204 = Concatenate Strings(w128, w132) -> (w133:string)
            n205 = String To Byte Array(string=w133) -> (unsigned byte array=w114:u8[])
            n206 = To Unsigned Long Integer(number=w114) -> (unsigned 32bit integer=w113:u32[])
            n207 = stacked-sequence {
              tunnel: enum16{"128", "192", "256", "auto"}."auto" ("Mode (auto)") -> [w611]
              tunnel: w113 -> [w616]
              tunnel: [w617] -> w121
              frame #0 {
                n208 = Array Size(array=w616) -> (size(s)=w612:i32)
                n209 = case shown="\"auto\", Par défaut" w611 {
                  tunnel: w612 -> [w626 _ _ _]
                  tunnel: [w627 16 24 32] -> w614
                  frame "auto", Default {
                    n210 = Less Or Equal?(x=w626, y=16) -> (x <= y?=w628:bool)
                    n211 = case shown="Faux" w628 {
                      tunnel: [w630 16] -> w627
                      tunnel: w626 -> [w633 _]
                      frame False {
                        n212 = Less Or Equal?(x=w633, y=24) -> (x <= y?=w631:bool)
                        n213 = case shown="Faux" w631 {
                          tunnel: [32 ("y") 24 ("y")] -> w630
                          frame False {
                          }
                          frame True {
                          }
                        }
                      }
                      frame True {
                      }
                    }
                  }
                  frame "128" {
                  }
                  frame "192" {
                  }
                  frame "256" {
                  }
                }
                n214 = Less?(x=w612, y=w614) -> (x < y?=w613:bool)
                n215 = case shown="Vrai" w613 {
                  tunnel: w616 -> [w620 w621]
                  tunnel: w614 -> [w619 w625]
                  tunnel: [w618 w623] -> w615
                  frame False {
                    # "Длина ключа\nбольше требуемой-\nотсекаем лишнее"
                    n216 = Array Subset(array=w620, length=w619) -> (w618:u32[])  [unwired: 1 in]
                  }
                  frame True {
                    # "Длина ключа\nменьше требуемой-\nдополняем нулями"
                    n217 = Initialize Array(u32 0, w625) -> (w624:u32[])
                    n218 = Replace Array Subset(array=w624, new element=w621) -> (w623:u32[])  [unwired: 1 in]
                  }
                }
                n219 = Array Size(array=w615) -> (size(s)=w610:i32)
                n220 = Logical Shift(y=i8 -2, x=w610) -> (x << y=w603:i32)
                n221 = case shown="8" w603 {
                  tunnel: [10 12 14] -> w600
                  frame 4, Default {
                  }
                  frame 6 {
                  }
                  frame 8 {
                  }
                }
                n222 = Increment(x=w600) -> (x+1=w601:i32)
                n223 = Multiply(x=4, y=w601) -> (x*y=w607:i32)
                n224 = Logical Shift(y=i8 2, x=w607) -> (x << y=w606:i32)
                n225 = Initialize Array(u32 0 ("element"), w606) -> (w608:u32[])
                n226 = Replace Array Subset(array=w608, new element=w615) -> (w609:u32[])  [unwired: 1 in]
                n227 = while {
                  tunnel: w607 -> [w692]
                  tunnel: w603 -> [w672]
                  shift-right: [w649] -> w617
                  shift-left: w609 -> [w673]
                  tunnel: w614 -> [w671]
                  i -> [w693]
                  stop <- w691 continue-if-true
                  n228 = Add(x=w672, y=w693) -> (x+y=w675:i32)
                  n229 = Less?(x=w675, y=w692) -> (x < y?=w691:bool)
                  n230 = Quotient & Remainder(x=w675, y=w672) -> (x-y*floor(x/y)=w680:i32, floor(x/y)=w674:i32)
                  n231 = Logical Shift(y=i8 2, x=w675) -> (x << y=w644:i32)
                  n232 = Equal To 0?(x=w680) -> (x = 0?=w681:bool)
                  n233 = Subtract(x=w644, y=4) -> (x-y=w685:i32)
                  n234 = Subtract(x=w644, y=3) -> (x-y=w684:i32)
                  n235 = Subtract(x=w644, y=2) -> (x-y=w683:i32)
                  n236 = Subtract(x=w644, y=1) -> (x-y=w682:i32)
                  n237 = Index Array(array=w673, index #1=w685, index #2=w684, index #3=w683, index #4=w682) -> (element #1=w679:u32, element #2=w678:u32, element #3=w677:u32, element #4=w676:u32)
                  n238 = case shown="Faux" w681 {
                    tunnel: w672 -> [w708 _]
                    tunnel: w680 -> [w706 _]
                    tunnel: w679 -> [w701 w734]
                    tunnel: w678 -> [w700 w733]
                    tunnel: w677 -> [w699 w732]
                    tunnel: w676 -> [w698 w731]
                    tunnel: w674 -> [_ w730]
                    tunnel: [w697 w727] -> w653
                    tunnel: [w696 w726] -> w652
                    tunnel: [w695 w725] -> w651
                    tunnel: [w694 w724] -> w650
                    frame False {
                      n239 = Greater?(x=w708, y=6) -> (0:w704:bool)
                      n240 = Equal?(x=w706, y=4) -> (x = y?=w703:bool)
                      n241 = And(x=w704, y=w703) -> (x .and. y?=w702:bool)
                      n242 = case shown="Faux" w702 {
                        tunnel: w701 -> [w712 w721]
                        tunnel: w700 -> [w711 w720]
                        tunnel: w699 -> [w710 w719]
                        tunnel: w698 -> [w709 w718]
                        tunnel: [w712 w717] -> w697
                        tunnel: [w711 w716] -> w696
                        tunnel: [w710 w715] -> w695
                        tunnel: [w709 w714] -> w694
                        frame False {
                        }
                        frame True {
                          # "Sbox"
                          n243 = Index Array(array=u32[] [99, 124, 119, 123, 242, 107, 111, 197, 48, 1, 103, 43, 254, 215, 171, 118, 202, 130, 201, 125, 250, 89, 71, 240, 173, 212, 162, 175, 156, 164, 114, 192, 183, 253, 147, 38, 54, 63, 247, 204, 52, 165, 229, 241, 113, 216, 49, 21, 4, 199, 35, 195, 24, 150, 5, 154, 7, 18, 128, 226, 235, 39, 178, 117, 9, 131, 44, 26, 27, 110, 90, 160, 82, 59, 214, 179, 41, 227, 47, 132, 83, 209, 0, 237, 32, 252, 177, 91, 106, 203, 190, 57, 74, 76, 88, 207, 208, 239, 170, 251, 67, 77, 51, 133, 69, 249, 2, 127, 80, 60, 159, 168, 81, 163, 64, 143, 146, 157, 56, 245, 188, 182, 218, 33, 16, 255, 243, 210, 205, 12, 19, 236, 95, 151, 68, 23, 196, 167, 126, 61, 100, 93, 25, 115, 96, 129, 79, 220, 34, 42, 144, 136, 70, 238, 184, 20, 222, 94, 11, 219, 224, 50, 58, 10, 73, 6, 36, 92, 194, 211, 172, 98, 145, 149, 228, 121, 231, 200, 55, 109, 141, 213, 78, 169, 108, 86, 244, 234, 101, 122, 174, 8, 186, 120, 37, 46, 28, 166, 180, 198, 232, 221, 116, 31, 75, 189, 139, 138, 112, 62, 181, 102, 72, 3, 246, 14, 97, 53, 87, 185, 134, 193, 29, 158, 225, 248, 152, 17, 105, 217, 142, 148, 155, 30, 135, 233, 206, 85, 40, 223, 140, 161, 137, 13, 191, 230, 66, 104, 65, 153, 45, 15, 176, 84, 187, 22] ("Sbox"), index #1=w721, index #2=w720, index #3=w719, index #4=w718) -> (element #1=w717:u32, element #2=w716:u32, element #3=w715:u32, element #4=w714:u32)
                        }
                      }
                    }
                    frame True {
                      # "Sbox"
                      # "Rcon"
                      n244 = Index Array(array=u32[] [0, 1, 2, 4, 8, 16, 32, 64, 128, 27, 54] ("Rcon"), index=w730) -> (element=w729:u32)
                      n245 = Index Array(array=u32[] [99, 124, 119, 123, 242, 107, 111, 197, 48, 1, 103, 43, 254, 215, 171, 118, 202, 130, 201, 125, 250, 89, 71, 240, 173, 212, 162, 175, 156, 164, 114, 192, 183, 253, 147, 38, 54, 63, 247, 204, 52, 165, 229, 241, 113, 216, 49, 21, 4, 199, 35, 195, 24, 150, 5, 154, 7, 18, 128, 226, 235, 39, 178, 117, 9, 131, 44, 26, 27, 110, 90, 160, 82, 59, 214, 179, 41, 227, 47, 132, 83, 209, 0, 237, 32, 252, 177, 91, 106, 203, 190, 57, 74, 76, 88, 207, 208, 239, 170, 251, 67, 77, 51, 133, 69, 249, 2, 127, 80, 60, 159, 168, 81, 163, 64, 143, 146, 157, 56, 245, 188, 182, 218, 33, 16, 255, 243, 210, 205, 12, 19, 236, 95, 151, 68, 23, 196, 167, 126, 61, 100, 93, 25, 115, 96, 129, 79, 220, 34, 42, 144, 136, 70, 238, 184, 20, 222, 94, 11, 219, 224, 50, 58, 10, 73, 6, 36, 92, 194, 211, 172, 98, 145, 149, 228, 121, 231, 200, 55, 109, 141, 213, 78, 169, 108, 86, 244, 234, 101, 122, 174, 8, 186, 120, 37, 46, 28, 166, 180, 198, 232, 221, 116, 31, 75, 189, 139, 138, 112, 62, 181, 102, 72, 3, 246, 14, 97, 53, 87, 185, 134, 193, 29, 158, 225, 248, 152, 17, 105, 217, 142, 148, 155, 30, 135, 233, 206, 85, 40, 223, 140, 161, 137, 13, 191, 230, 66, 104, 65, 153, 45, 15, 176, 84, 187, 22] ("Sbox"), index #1=w733, index #2=w732, index #3=w731, index #4=w734) -> (element #1=w728:u32, element #2=w726:u32, element #3=w725:u32, element #4=w724:u32)
                      n246 = Exclusive Or(1:w728, 2:w729) -> (0:w727:u32)
                    }
                  }
                  n247 = Subtract(x=w644, y=w671) -> (x-y=w670:i32)
                  n248 = Add(x=w670, y=0) -> (x+y=w665:i32)
                  n249 = Add(x=w670, y=1) -> (x+y=w664:i32)
                  n250 = Add(x=w670, y=2) -> (x+y=w663:i32)
                  n251 = Add(x=w670, y=3) -> (x+y=w662:i32)
                  n252 = Index Array(array=w673, index #1=w665, index #2=w664, index #3=w663, index #4=w662) -> (element #1=w661:u32, element #2=w660:u32, element #3=w659:u32, element #4=w658:u32)
                  n253 = Exclusive Or(1:w653, 2:w661) -> (0:w657:u32)
                  n254 = Exclusive Or(1:w652, 2:w660) -> (0:w656:u32)
                  n255 = Exclusive Or(1:w651, 2:w659) -> (0:w655:u32)
                  n256 = Exclusive Or(1:w650, 2:w658) -> (0:w654:u32)
                  n257 = Add(x=w644, y=0) -> (x+y=w643:i32)
                  n258 = Add(x=w644, y=1) -> (x+y=w642:i32)
                  n259 = Add(x=w644, y=2) -> (x+y=w641:i32)
                  n260 = Add(x=w644, y=3) -> (x+y=w640:i32)
                  n261 = Replace Array Subset(array=w673, new element #1=w657, index #1=w643, new element #2=w656, index #2=w642, new element #3=w655, index #3=w641, new element #4=w654, index #4=w640) -> (w649:u32[])
                }
              }
            }
          }
          frame "MixBlocks" {
            n262 = for {
              N: w742 -> [w765]
              shift-right: [w767] -> _
              shift-left: w748 -> [w768]
              shift-right: [w751] -> _
              shift-left: w740 -> [w766]
              shift-right: [w756] -> _
              shift-left: w747 -> [w764]
              tunnel: w745 -> [w763]
              shift-right: [w762] -> _
              shift-left: _ -> [w761]
              shift-right: [w760] -> _
              shift-left: _ -> [w759]
              shift-right: [w758] -> _
              shift-left: _ -> [w757]
              shift-right: [w755] -> _
              shift-left: _ -> [w754]
              shift-right: [w753] -> w749
              shift-left: "" -> [w752]
              i -> [w769]
              # "> cipherTxt >"
              # "> cipherCntr >"
              # "> blockLength >"
              # "> cipherChar >"
              # "> cipherCharStr >"
              # "> PlainText >"
              # "> blockSize >"
              # "> keySchedule >"
              # "> counterBlock >"
              # "b"
              n263 = while {
                shift-right: [w791] -> _
                shift-left: "Mix Bytes Phases" -> [w792]
                tunnel: w769 -> [w789]
                shift-right: [w787] -> w767
                shift-left: w768 -> [w788]
                shift-right: [w784] -> w751
                shift-left: w766 -> [w786]
                tunnel: w765 -> [w785]
                shift-right: [w771] -> w756
                shift-left: w764 -> [w783]
                tunnel: w763 -> [w782]
                shift-right: [w781] -> w762
                shift-left: w761 -> [w772]
                shift-right: [w780] -> w760
                shift-left: w759 -> [w777]
                shift-right: [w779] -> w758
                shift-left: w757 -> [w778]
                shift-right: [w776] -> w755
                shift-left: w754 -> [w775]
                shift-right: [w774] -> w753
                shift-left: w752 -> [w773]
                stop <- w790 stop-if-true
                n264 = case shown="\"Cipher Blocks\"" w792 {
                  tunnel: [T1."Cipher Blocks" ("Mix Bytes Phases") T1."Replace ciphered" ("Mix Bytes Phases") T1."Combine parts" ("Mix Bytes Phases") T1."Replace Blocks" ("Mix Bytes Phases")] -> w791
                  tunnel: [FALSE FALSE FALSE TRUE] -> w790
                  tunnel: w789 -> [w802 w835 w1181 _]
                  tunnel: w788 -> [w801 w828 w1172 w1201]
                  tunnel: [w800 w828 w1172 w1201] -> w787
                  tunnel: w786 -> [w799 w827 w1171 w1200]
                  tunnel: w785 -> [_ w834 _ _]
                  tunnel: [w799 w827 w1171 w1200] -> w784
                  tunnel: w783 -> [w795 w826 w1173 w1199]
                  tunnel: w782 -> [_ w833 w1178 _]
                  tunnel: [string[] [] w832 w1176 w1204] -> w781
                  tunnel: [i32[] [] w831 w1177 w1203] -> w780
                  tunnel: [0 ("blockSize") w830 w1174 w1198] -> w779
                  tunnel: w778 -> [_ _ w1180 w1198]
                  tunnel: w777 -> [_ _ w1179 w1203]
                  tunnel: [u16[] [] ("Cypher.Output") w829 w1175 w1202] -> w776
                  tunnel: w775 -> [_ _ w1175 w1202]
                  tunnel: [w793 w825 w1170 w1206] -> w774
                  tunnel: w773 -> [w793 w825 w1170 w1205]
                  tunnel: w772 -> [_ _ w1176 w1204]
                  tunnel: [w795 w826 w1173 w1199] -> w771
                  frame "Replace Blocks", Default {
                    n265 = for {
                      N: 4 -> [_]
                      tunnel: w802 -> [w820]
                      tunnel: w802 -> [w813]
                      shift-right: [w806] -> w800
                      shift-left: w801 -> [w807]
                      i -> [w819]
                      # "c"
                      n266 = Divide(x=w813, y="0x100000000") -> (x/y=w811:dbl)
                      n267 = Multiply(x=-8, y=w819) -> (x*y=w812:i32)
                      n268 = Logical Shift(y=w812, x=w820) -> (x << y=w822:i32)
                      n269 = And(x=w822, y=u16 255 ("0xff")) -> (x .and. y?=w817:i32)
                      n270 = Subtract(x=15, y=w819) -> (x-y=w816:i32)
                      n271 = Logical Shift(y=w812, x=w811) -> (x << y=w810:u32)
                      n272 = Subtract(x=w816, y=4) -> (x-y=w814:i32)
                      n273 = Replace Array Subset(array=w807, new element #1=w817, index #1=w816, new element #2=w810, index #2=w814) -> (w806:u32[])
                    }
                  }
                  frame "Cipher Blocks" {
                    n274 = Decrement(x=w834) -> (x-1=w836:i32)
                    n275 = Greater?(x=w836, y=w835) -> (0:w837:bool)
                    n276 = String Length(string=w833) -> (length=w839:i32)
                    n277 = Decrement(x=w839) -> (x-1=w838:i32)
                    n278 = stacked-sequence {
                      tunnel: w828 -> [w848]
                      tunnel: [w849] -> w829
                      tunnel: w827 -> [w847]
                      tunnel: errorcluster {"status"=FALSE, "code"=0, "source"=""} ("error in") -> [w845]
                      tunnel: [w846] -> _
                      frame #0 {
                        n279 = case shown="Pas d'erreur" w845 {
                          selector: w845 -> [_ w1168]
                          tunnel: [_ w1168] -> w846
                          tunnel: w847 -> [w854 _]
                          tunnel: w848 -> [w853 _]
                          tunnel: [w852 u16[] []] -> w849
                          tunnel: 4 ("Nb") -> [w851 _]
                          frame No Error {
                            n280 = while {
                              shift-right: [w858] -> _
                              shift-left: enum16{"Init", "Mix rows"}."Init" ("Cipher Phases") -> [w870]
                              tunnel: w854 -> [w869]
                              tunnel: w853 -> [w868]
                              shift-right: [w867] -> _
                              shift-left: _ -> [w866]
                              shift-right: [w865] -> _
                              shift-left: _ -> [w864]
                              shift-right: [w863] -> _
                              shift-left: _ -> [w862]
                              shift-right: [w861] -> _
                              shift-left: _ -> [w860]
                              tunnel: [w859] -> w852
                              tunnel: w851 -> [w856]
                              stop <- w857 stop-if-true
                              # "> Nr >"
                              # "> Nb >"
                              # "> State >"
                              # "> ExpandedKez(w)(2D) >"
                              n281 = case shown="\"Init\", Par défaut" w870 {
                                tunnel: w869 -> [w883 _]
                                tunnel: w868 -> [w881 _]
                                tunnel: [w878 w931] -> w867
                                tunnel: w866 -> [_ w931]
                                tunnel: [w877 w924] -> w865
                                tunnel: w864 -> [_ w925]
                                tunnel: [w871 w932] -> w863
                                tunnel: w862 -> [_ w932]
                                tunnel: [w875 w930] -> w861
                                tunnel: w860 -> [_ w930]
                                tunnel: [_ w927] -> w859
                                tunnel: [enum16{"Init", "Mix rows"}."Mix rows" ("Cipher Phases") _] -> w858
                                tunnel: [FALSE TRUE] -> w857
                                tunnel: w856 -> [w871 _]
                                frame "Init", Default {
                                # "> Nb >"
                                # "> ExpandedKey(w)(2D) >"
                                # "> Nr >"
                                n282 = Reshape Array(w883, 60 ("dimension size"), 4 ("dimension size")) -> (w878:u32[][])
                                n283 = for {
                                N: 16 -> [_]
                                tunnel: w881 -> [w918]
                                shift-right: [w916] -> w879
                                shift-left: u16[][] [[0, 0, 0, 0], [0, 0, 0, 0], [0, 0, 0, 0], [0, 0, 0, 0]] ("State.Out") -> [w917]
                                i -> [w923]
                                n284 = Quotient & Remainder(x=w923, y=4) -> (x-y*floor(x/y)=w920:i32, floor(x/y)=w919:i32)
                                n285 = Index Array(array=w918, index=w923) -> (element=w921:u32)
                                n286 = Replace Array Subset(array=w917, new element=w921, index (row)=w920, index (col)=w919) -> (w916:u16[][])
                                }
                                n287 = Array Size(array=w878) -> (size(s)=w884:i32[])
                                n288 = Index Array(array=w884, index=0) -> (element=w887:i32)
                                n289 = Divide(x=w887, y=w871) -> (x/y=w886:dbl)
                                n290 = Decrement(x=w886) -> (x-1=w876:dbl)
                                n291 = To Long Integer(number=w876) -> (32bit integer=w875:i32)
                                n292 = stacked-sequence {
                                tunnel: w878 -> [w890]
                                tunnel: w871 -> [w892]
                                tunnel: w879 -> [w894]
                                tunnel: [w895] -> w877
                                tunnel: 0 ("rnd (0)") -> [w893]
                                frame #0 {
                                n293 = for {
                                N: 4 -> [_]
                                tunnel: w894 -> [w901]
                                tunnel: w890 -> [w900]
                                tunnel: w892 -> [w899]
                                tunnel: w893 -> [w898]
                                shift-right: [w896] -> w895
                                shift-left: w894 -> [w897]
                                i -> [w902]
                                # "w"
                                # "state"
                                # "r"
                                n294 = for {
                                N: w899 -> [_]
                                tunnel: w902 -> [w907]
                                tunnel: w901 -> [w910]
                                tunnel: w900 -> [w915]
                                tunnel: w898 -> [w914]
                                shift-right: [w903] -> w896
                                shift-left: w897 -> [w904]
                                i -> [w906]
                                # "c"
                                n295 = Multiply(x=w914, y=4) -> (x*y=w912:i32)
                                n296 = Add(x=w912, y=w906) -> (x+y=w911:i32)
                                n297 = Index Array(array=w910, index (row)=w907, index (col)=w906) -> (element=w909:u16)
                                n298 = Index Array(array=w915, index (row)=w911, index (col)=w907) -> (element=w908:u32)
                                n299 = Exclusive Or(1:w908, 2:w909) -> (0:w905:u32)
                                n300 = Replace Array Subset(array=w904, new element=w905, index (row)=w907, index (col)=w906) -> (w903:u16[][])
                                }
                                }
                                }
                                }
                                }
                                frame "Mix rows" {
                                # "var output : Array = new Array(4 * Nb); \n\tfor (var i : int = 0;i < 4 * Nb;i++)\n   {\n    output[i] = state[i % 4][Math.floor(i / 4)];\n\t\t\t}"
                                n301 = Decrement(x=w930) -> (x-1=w938:i32)
                                n302 = for {
                                N: w938 -> [_]
                                shift-right: [w1021] -> w933
                                shift-left: w925 -> [w1022]
                                tunnel: w932 -> [w1020]
                                tunnel: w931 -> [w1019]
                                i -> [w1024]
                                # "round"
                                n303 = stacked-sequence {
                                tunnel: w1020 -> [w1028]
                                tunnel: w1022 -> [w1030]
                                tunnel: [w1031] -> w1027
                                frame #0 {
                                n304 = for {
                                N: 4 -> [_]
                                tunnel: w1030 -> [w1035]
                                shift-right: [w1032] -> w1031
                                shift-left: w1030 -> [w1034]
                                tunnel: w1028 -> [w1033]
                                i -> [w1036]
                                # "> State.In >"
                                # "> State.Temp >"
                                # "r"
                                n305 = for {
                                N: w1033 -> [_]
                                tunnel: w1035 -> [w1044]
                                tunnel: w1036 -> [w1041]
                                shift-right: [w1037] -> w1032
                                shift-left: w1034 -> [w1038]
                                i -> [w1040]
                                # "Sbox"
                                # "s[r][c]"
                                # "c"
                                n306 = Index Array(array=w1044, index (row)=w1040, index (col)=w1041) -> (element=w1043:u16)
                                n307 = Index Array(array=u16[] [99, 124, 119, 123, 242, 107, 111, 197, 48, 1, 103, 43, 254, 215, 171, 118, 202, 130, 201, 125, 250, 89, 71, 240, 173, 212, 162, 175, 156, 164, 114, 192, 183, 253, 147, 38, 54, 63, 247, 204, 52, 165, 229, 241, 113, 216, 49, 21, 4, 199, 35, 195, 24, 150, 5, 154, 7, 18, 128, 226, 235, 39, 178, 117, 9, 131, 44, 26, 27, 110, 90, 160, 82, 59, 214, 179, 41, 227, 47, 132, 83, 209, 0, 237, 32, 252, 177, 91, 106, 203, 190, 57, 74, 76, 88, 207, 208, 239, 170, 251, 67, 77, 51, 133, 69, 249, 2, 127, 80, 60, 159, 168, 81, 163, 64, 143, 146, 157, 56, 245, 188, 182, 218, 33, 16, 255, 243, 210, 205, 12, 19, 236, 95, 151, 68, 23, 196, 167, 126, 61, 100, 93, 25, 115, 96, 129, 79, 220, 34, 42, 144, 136, 70, 238, 184, 20, 222, 94, 11, 219, 224, 50, 58, 10, 73, 6, 36, 92, 194, 211, 172, 98, 145, 149, 228, 121, 231, 200, 55, 109, 141, 213, 78, 169, 108, 86, 244, 234, 101, 122, 174, 8, 186, 120, 37, 46, 28, 166, 180, 198, 232, 221, 116, 31, 75, 189, 139, 138, 112, 62, 181, 102, 72, 3, 246, 14, 97, 53, 87, 185, 134, 193, 29, 158, 225, 248, 152, 17, 105, 217, 142, 148, 155, 30, 135, 233, 206, 85, 40, 223, 140, 161, 137, 13, 191, 230, 66, 104, 65, 153, 45, 15, 176, 84, 187, 22] ("Sbox"), index=w1043) -> (element=w1042:u16)
                                n308 = Replace Array Subset(array=w1038, new element=w1042, index (row)=w1040, index (col)=w1041) -> (w1037:u16[][])
                                }
                                }
                                }
                                }
                                n309 = Increment(x=w1024) -> (x+1=w1023:i32)
                                n310 = stacked-sequence {
                                tunnel: w1020 -> [w1045]
                                tunnel: w1027 -> [w1047]
                                tunnel: [w1048] -> w1026
                                frame #0 {
                                n311 = for {
                                N: 3 -> [_]
                                tunnel: w1047 -> [w1058]
                                shift-right: [w1054] -> w1048
                                shift-left: w1047 -> [w1055]
                                tunnel: w1045 -> [w1049]
                                i -> [w1057]
                                # "> t[c] >"
                                # "> State.In >"
                                # "> State.Temp >"
                                # "r"
                                n312 = Increment(x=w1057) -> (x+1=w1056:i32)
                                n313 = for {
                                N: 4 -> [_]
                                tunnel: w1058 -> [w1073]
                                tunnel: w1056 -> [w1069]
                                shift-right: [w1065] -> w1052
                                shift-left: i32[] [0, 0, 0, 0] ("t[c]") -> [w1066]
                                tunnel: w1049 -> [w1071]
                                i -> [w1068]
                                # "c"
                                n314 = Add(x=w1069, y=w1068) -> (x+y=w1072:i32)
                                n315 = Quotient & Remainder(x=w1072, y=w1071) -> (x-y*floor(x/y)=w1070:i32)  [unwired: 1 out]
                                n316 = Index Array(array=w1073, index (row)=w1069, index (col)=w1070) -> (element=w1067:u16)
                                n317 = Insert Into Array(array=w1066, index=w1068, new element=w1067) -> (w1065:i32[])
                                }
                                n318 = for {
                                N: 4 -> [_]
                                tunnel: w1056 -> [w1064]
                                shift-right: [w1060] -> w1054
                                shift-left: w1055 -> [w1061]
                                tunnel: w1052 -> [w1059]
                                i -> [w1063]
                                # "c"
                                n319 = Index Array(array=w1059, index=w1063) -> (element=w1062:i32)
                                n320 = Replace Array Subset(array=w1061, new element=w1062, index (row)=w1064, index (col)=w1063) -> (w1060:u16[][])
                                }
                                }
                                }
                                }
                                n321 = stacked-sequence {
                                tunnel: w1026 -> [w1075]
                                tunnel: [w1076] -> w1025
                                frame #0 {
                                n322 = for {
                                N: 4 -> [_]
                                shift-right: [w1120] -> w1076
                                shift-left: w1075 -> [w1121]
                                tunnel: w1075 -> [w1122]
                                i -> [w1123]
                                # "> b >"
                                # "> a >"
                                # "> State.In >"
                                # "> State.Temp >"
                                # "c"
                                n323 = To Unsigned Word Integer(number=i32[] [0, 0, 0, 0] ("t[c]")) -> (unsigned 16bit integer=w1117:u16[])
                                n324 = To Unsigned Word Integer(number=i32[] [0, 0, 0, 0] ("t[c]")) -> (unsigned 16bit integer=w1116:u16[])
                                n325 = for {
                                N: 4 -> [_]
                                tunnel: w1122 -> [w1140]
                                tunnel: w1123 -> [w1139]
                                shift-right: [w1126] -> w1115
                                shift-left: w1117 -> [w1127]
                                shift-right: [w1124] -> w1114
                                shift-left: w1116 -> [w1125]
                                i -> [w1138]
                                # "s[i][c]"
                                # "i"
                                n326 = Index Array(array=w1140, index (row)=w1138, index (col)=w1139) -> (element=w1132:u16)
                                n327 = And(x=w1132, y=u16 128 ("0x80")) -> (x .and. y?=w1135:u16)
                                n328 = Logical Shift(y=i8 1, x=w1132) -> (x << y=w1129:u16)
                                n329 = Number To Boolean Array(number=w1135) -> (Boolean array=w1134:bool[])
                                n330 = Insert Into Array(array=w1127, index=w1138, new element=w1132) -> (w1126:u16[])
                                n331 = Exclusive Or(1:u16 283 ("0x011b"), 2:w1129) -> (0:w1130:u16)
                                n332 = Or Array Elements(Boolean array=w1134) -> (logical OR=w1133:bool)
                                n333 = Select(t=w1130, s=w1133, f=w1129) -> (s? t:f=w1137:u16)
                                n334 = Insert Into Array(array=w1125, index=w1138, new element=w1137) -> (w1124:u16[])
                                }
                                n335 = Index Array(array=w1114, index #1=0 ("index"), index #2=1 ("index"), index #3=2 ("index"), index #4=3 ("index")) -> (element #1=w1085:u16, element #2=w1097:u16, element #3=w1092:u16, element #4=w1082:u16)
                                n336 = Index Array(array=w1115, index #1=0 ("index"), index #2=1 ("index"), index #3=2 ("index"), index #4=3 ("index")) -> (element #1=w1086:u16, element #2=w1084:u16, element #3=w1083:u16, element #4=w1091:u16)
                                n337 = Exclusive Or(1:w1084, 2:w1085) -> (0:w1104:u16)
                                n338 = Exclusive Or(1:w1097, 2:w1104) -> (0:w1103:u16)
                                n339 = Exclusive Or(1:w1084, 2:w1086) -> (0:w1095:u16)
                                n340 = Exclusive Or(1:w1083, 2:w1103) -> (0:w1102:u16)
                                n341 = Exclusive Or(1:w1085, 2:w1086) -> (0:w1089:u16)
                                n342 = Exclusive Or(1:w1097, 2:w1086) -> (0:w1100:u16)
                                n343 = Exclusive Or(1:w1092, 2:w1095) -> (0:w1094:u16)
                                n344 = Exclusive Or(1:w1091, 2:w1102) -> (0:w1101:u16)
                                n345 = Exclusive Or(1:w1084, 2:w1089) -> (0:w1088:u16)
                                n346 = Exclusive Or(1:w1083, 2:w1100) -> (0:w1099:u16)
                                n347 = Exclusive Or(1:w1091, 2:w1094) -> (0:w1093:u16)
                                n348 = Exclusive Or(1:w1083, 2:w1088) -> (0:w1087:u16)
                                n349 = Exclusive Or(1:w1092, 2:w1099) -> (0:w1098:u16)
                                n350 = Exclusive Or(1:w1082, 2:w1093) -> (0:w1090:u16)
                                n351 = Exclusive Or(1:w1082, 2:w1087) -> (0:w1081:u16)
                                n352 = Exclusive Or(1:w1091, 2:w1098) -> (0:w1096:u16)
                                n353 = Replace Array Subset(array=w1121, new element #1=w1101, index (row) #1=0 ("disabled index (col)"), index (col) #1=w1123, new element #2=w1096, index (row) #2=1 ("disabled index (col)"), index (col) #2=w1123, new element #3=w1090, index (row) #3=2 ("disabled index (col)"), index (col) #3=w1123, new element #4=w1081, index (row) #4=3 ("disabled index (col)"), index (col) #4=w1123) -> (w1120:u16[][])
                                }
                                }
                                }
                                n354 = stacked-sequence {
                                tunnel: w1019 -> [w1141]
                                tunnel: w1020 -> [w1143]
                                tunnel: w1025 -> [w1145]
                                tunnel: [w1146] -> w1021
                                tunnel: w1023 -> [w1144]
                                frame #0 {
                                n355 = for {
                                N: 4 -> [_]
                                tunnel: w1145 -> [w1152]
                                tunnel: w1141 -> [w1151]
                                tunnel: w1143 -> [w1150]
                                tunnel: w1144 -> [w1149]
                                shift-right: [w1147] -> w1146
                                shift-left: w1145 -> [w1148]
                                i -> [w1153]
                                # "w"
                                # "state"
                                # "r"
                                n356 = for {
                                N: w1150 -> [_]
                                tunnel: w1153 -> [w1158]
                                tunnel: w1152 -> [w1161]
                                tunnel: w1151 -> [w1166]
                                tunnel: w1149 -> [w1165]
                                shift-right: [w1154] -> w1147
                                shift-left: w1148 -> [w1155]
                                i -> [w1157]
                                # "c"
                                n357 = Multiply(x=w1165, y=4) -> (x*y=w1163:i32)
                                n358 = Add(x=w1163, y=w1157) -> (x+y=w1162:i32)
                                n359 = Index Array(array=w1161, index (row)=w1158, index (col)=w1157) -> (element=w1160:u16)
                                n360 = Index Array(array=w1166, index (row)=w1162, index (col)=w1158) -> (element=w1159:u32)
                                n361 = Exclusive Or(1:w1159, 2:w1160) -> (0:w1156:u32)
                                n362 = Replace Array Subset(array=w1155, new element=w1156, index (row)=w1158, index (col)=w1157) -> (w1154:u16[][])
                                }
                                }
                                }
                                }
                                }
                                n363 = stacked-sequence {
                                tunnel: w932 -> [w994]
                                tunnel: w933 -> [w996]
                                tunnel: [w997] -> w937
                                frame #0 {
                                n364 = for {
                                N: 4 -> [_]
                                tunnel: w996 -> [w1001]
                                shift-right: [w998] -> w997
                                shift-left: w996 -> [w1000]
                                tunnel: w994 -> [w999]
                                i -> [w1002]
                                # "> State.In >"
                                # "> State.Temp >"
                                # "r"
                                n365 = for {
                                N: w999 -> [_]
                                tunnel: w1001 -> [w1010]
                                tunnel: w1002 -> [w1007]
                                shift-right: [w1003] -> w998
                                shift-left: w1000 -> [w1004]
                                i -> [w1006]
                                # "Sbox"
                                # "s[r][c]"
                                # "c"
                                n366 = Index Array(array=w1010, index (row)=w1006, index (col)=w1007) -> (element=w1009:u16)
                                n367 = Index Array(array=u16[] [99, 124, 119, 123, 242, 107, 111, 197, 48, 1, 103, 43, 254, 215, 171, 118, 202, 130, 201, 125, 250, 89, 71, 240, 173, 212, 162, 175, 156, 164, 114, 192, 183, 253, 147, 38, 54, 63, 247, 204, 52, 165, 229, 241, 113, 216, 49, 21, 4, 199, 35, 195, 24, 150, 5, 154, 7, 18, 128, 226, 235, 39, 178, 117, 9, 131, 44, 26, 27, 110, 90, 160, 82, 59, 214, 179, 41, 227, 47, 132, 83, 209, 0, 237, 32, 252, 177, 91, 106, 203, 190, 57, 74, 76, 88, 207, 208, 239, 170, 251, 67, 77, 51, 133, 69, 249, 2, 127, 80, 60, 159, 168, 81, 163, 64, 143, 146, 157, 56, 245, 188, 182, 218, 33, 16, 255, 243, 210, 205, 12, 19, 236, 95, 151, 68, 23, 196, 167, 126, 61, 100, 93, 25, 115, 96, 129, 79, 220, 34, 42, 144, 136, 70, 238, 184, 20, 222, 94, 11, 219, 224, 50, 58, 10, 73, 6, 36, 92, 194, 211, 172, 98, 145, 149, 228, 121, 231, 200, 55, 109, 141, 213, 78, 169, 108, 86, 244, 234, 101, 122, 174, 8, 186, 120, 37, 46, 28, 166, 180, 198, 232, 221, 116, 31, 75, 189, 139, 138, 112, 62, 181, 102, 72, 3, 246, 14, 97, 53, 87, 185, 134, 193, 29, 158, 225, 248, 152, 17, 105, 217, 142, 148, 155, 30, 135, 233, 206, 85, 40, 223, 140, 161, 137, 13, 191, 230, 66, 104, 65, 153, 45, 15, 176, 84, 187, 22] ("Sbox"), index=w1009) -> (element=w1008:u16)
                                n368 = Replace Array Subset(array=w1004, new element=w1008, index (row)=w1006, index (col)=w1007) -> (w1003:u16[][])
                                }
                                }
                                }
                                }
                                n369 = stacked-sequence {
                                tunnel: w932 -> [w965]
                                tunnel: w937 -> [w967]
                                tunnel: [w968] -> w936
                                frame #0 {
                                n370 = for {
                                N: 3 -> [_]
                                tunnel: w967 -> [w978]
                                shift-right: [w974] -> w968
                                shift-left: w967 -> [w975]
                                tunnel: w965 -> [w969]
                                i -> [w977]
                                # "> t[c] >"
                                # "> State.In >"
                                # "> State.Temp >"
                                # "r"
                                n371 = Increment(x=w977) -> (x+1=w976:i32)
                                n372 = for {
                                N: 4 -> [_]
                                tunnel: w978 -> [w993]
                                tunnel: w976 -> [w989]
                                shift-right: [w985] -> w972
                                shift-left: i32[] [0, 0, 0, 0] ("t[c]") -> [w986]
                                tunnel: w969 -> [w991]
                                i -> [w988]
                                # "c"
                                n373 = Add(x=w989, y=w988) -> (x+y=w992:i32)
                                n374 = Quotient & Remainder(x=w992, y=w991) -> (x-y*floor(x/y)=w990:i32)  [unwired: 1 out]
                                n375 = Index Array(array=w993, index (row)=w989, index (col)=w990) -> (element=w987:u16)
                                n376 = Insert Into Array(array=w986, index=w988, new element=w987) -> (w985:i32[])
                                }
                                n377 = for {
                                N: 4 -> [_]
                                tunnel: w976 -> [w984]
                                shift-right: [w980] -> w974
                                shift-left: w975 -> [w981]
                                tunnel: w972 -> [w979]
                                i -> [w983]
                                # "c"
                                n378 = Index Array(array=w979, index=w983) -> (element=w982:i32)
                                n379 = Replace Array Subset(array=w981, new element=w982, index (row)=w984, index (col)=w983) -> (w980:u16[][])
                                }
                                }
                                }
                                }
                                n380 = stacked-sequence {
                                tunnel: w931 -> [w939]
                                tunnel: w932 -> [w941]
                                tunnel: w936 -> [w943]
                                tunnel: [w944] -> w924
                                tunnel: w930 -> [w942]
                                frame #0 {
                                n381 = for {
                                N: 4 -> [_]
                                tunnel: w943 -> [w950]
                                tunnel: w939 -> [w949]
                                tunnel: w941 -> [w948]
                                tunnel: w942 -> [w947]
                                shift-right: [w945] -> w944
                                shift-left: w943 -> [w946]
                                i -> [w951]
                                # "w"
                                # "state"
                                # "r"
                                n382 = for {
                                N: w948 -> [_]
                                tunnel: w951 -> [w956]
                                tunnel: w950 -> [w959]
                                tunnel: w949 -> [w964]
                                tunnel: w947 -> [w963]
                                shift-right: [w952] -> w945
                                shift-left: w946 -> [w953]
                                i -> [w955]
                                # "c"
                                n383 = Multiply(x=w963, y=4) -> (x*y=w961:i32)
                                n384 = Add(x=w961, y=w955) -> (x+y=w960:i32)
                                n385 = Index Array(array=w959, index (row)=w956, index (col)=w955) -> (element=w958:u16)
                                n386 = Index Array(array=w964, index (row)=w960, index (col)=w956) -> (element=w957:u32)
                                n387 = Exclusive Or(1:w957, 2:w958) -> (0:w954:u32)
                                n388 = Replace Array Subset(array=w953, new element=w954, index (row)=w956, index (col)=w955) -> (w952:u16[][])
                                }
                                }
                                }
                                }
                                n389 = Multiply(x=4, y=w932) -> (x*y=w929:i32)
                                n390 = Initialize Array(u16 0 ("x"), w929) -> (w928:u16[])
                                n391 = for {
                                N: w929 -> [_]
                                shift-right: [w1011] -> w927
                                shift-left: w928 -> [w1012]
                                tunnel: w924 -> [w1013]
                                i -> [w1015]
                                n392 = Quotient & Remainder(x=w1015, y=4) -> (x-y*floor(x/y)=w1017:i32, floor(x/y)=w1016:i32)
                                n393 = Index Array(array=w1013, index (row)=w1017, index (col)=w1016) -> (element=w1014:u16)
                                n394 = Replace Array Subset(array=w1012, new element=w1014, index=w1015) -> (w1011:u16[])
                                }
                                }
                              }
                            }
                          }
                          frame Error {
                          }
                        }
                      }
                    }
                    "cipherCntr" <- w829
                    n395 = Quotient & Remainder(x=w838, y=w826) -> (x-y*floor(x/y)=w840:i32)  [unwired: 1 out]
                    n396 = Increment(x=w840) -> (x+1=w841:i32)
                    n397 = Select(t=w826, s=w837, f=w841) -> (s? t:f=w830:i32)
                    "blockLength" <- w830
                    n398 = Initialize Array("", w830) -> (w832:string[])
                    "cipherCharStr" <- w832
                    n399 = Initialize Array(0, w830) -> (w831:i32[])
                    "cipherChar" <- w831
                  }
                  frame "Replace ciphered" {
                    n400 = for {
                      N: w1180 -> [w1183]
                      tunnel: w1181 -> [w1194]
                      shift-right: [w1187] -> w1177
                      shift-left: w1179 -> [w1188]
                      tunnel: w1173 -> [w1186]
                      tunnel: w1178 -> [w1185]
                      tunnel: w1175 -> [w1184]
                      tunnel: [w1183] -> w1174
                      i -> [w1190]
                      n401 = Multiply(x=w1186, y=w1194) -> (x*y=w1193:i32)
                      n402 = Add(x=w1190, y=w1193) -> (x+y=w1192:i32)
                      n403 = String To Byte Array(string=w1185) -> (unsigned byte array=w1195:u8[])
                      n404 = Index Array(array=w1195, index=w1192) -> (element=w1191:u8)
                      n405 = Index Array(array=w1184, index=w1190) -> (element=w1196:u16)
                      n406 = Exclusive Or(1:w1191, 2:w1196) -> (0:w1189:u16)
                      n407 = Replace Array Subset(array=w1188, new element=w1189, index=w1190) -> (w1187:i32[])
                    }
                  }
                  frame "Combine parts" {
                    n408 = Byte Array To String(unsigned byte array=w1203) -> (string=w1207:string)
                    n409 = Concatenate Strings(w1205, w1207) -> (w1206:string)
                  }
                }
              }
            }
          }
          frame "ToB64" {
            n410 = Concatenate Strings(w1212, w1211) -> (w1223:string)
            n411 = stacked-sequence {
              tunnel: "\n" ("Line separator (\\n)") -> [w1244]
              tunnel: w1223 -> [w1226]
              tunnel: [w1243] -> w1221
              frame #0 {
                w1236 = u8[] [65, 66, 67, 68, 69, 70, 71, 72, 73, 74, 75, 76, 77, 78, 79, 80, 81, 82, 83, 84, 85, 86, 87, 88, 89, 90, 97, 98, 99, 100, 101, 102, 103, 104, 105, 106, 107, 108, 109, 110, 111, 112, 113, 114, 115, 116, 117, 118, 119, 120, 121, 122, 48, 49, 50, 51, 52, 53, 54, 55, 56, 57, 43, 47]  # B64 Map
                w1230 = 3 ("y")
                n412 = String Length(string=w1226) -> (length=w1229:i32)
                n413 = Quotient & Remainder(x=w1229, y=w1230) -> (x-y*floor(x/y)=w1231:i32)  [unwired: 1 out]
                n414 = Subtract(x=w1230, y=w1231) -> (x-y=w1234:i32)
                n415 = Greater Than 0?(x=w1231) -> (x > 0?=w1232:bool)
                n416 = Select(t=w1234, s=w1232, f=0 ("y")) -> (s? t:f=w1239:i32)
                n417 = String Subset(string="\u0000\u0000\u0000\u0000", length (rest)=w1239) -> (substring=w1225:string)  [unwired: 1 in]
                n418 = Concatenate Strings(w1226, w1225) -> (w1227:string)
                n419 = Type Cast(type=cluster{"u8":u8, "u8":u8, "u8":u8}[] [], x=w1227) -> (*(type *) &x=w1235:cluster{"u8":u8, "u8":u8, "u8":u8}[])
                n420 = for {
                  tunnel: w1235 -> [w1262] mode=indexing
                  tunnel: w1236 -> [w1256]
                  tunnel: w1244 -> [w1249]
                  tunnel: [w1247] -> w1245 mode=indexing
                  i -> [w1252]
                  w1253 = 15 ("x")
                  w1261 = 0  # I32
                  n421 = Type Cast(type=w1261, x=w1262) -> (*(type *) &x=w1260:i32)
                  n422 = And(x=w1252, y=w1253) -> (x .and. y?=w1254:i32)
                  n423 = for {
                    N: 4 -> [_]
                    shift-right: [w1270] -> _
                    shift-left: w1260 -> [w1267]
                    tunnel: [w1266] -> w1257 mode=indexing
                    n424 = Logical Shift(y=6, x=w1267) -> (x << y=w1270:i32)
                    n425 = Logical Shift(y=-26, x=w1267) -> (x << y=w1266:i32)
                  }
                  n426 = Less?(x=w1254, y=w1253) -> (x < y?=w1251:bool)
                  n427 = Select(t="", s=w1251, f=w1249) -> (s? t:f=w1248:string)
                  n428 = for {
                    tunnel: w1257 -> [w1265] mode=indexing
                    tunnel: w1256 -> [w1264]
                    tunnel: [w1263] -> w1255 mode=indexing
                    n429 = Index Array(array=w1264, index=w1265) -> (element=w1263:u8)
                  }
                  n430 = Byte Array To String(unsigned byte array=w1255) -> (string=w1259:string)
                  n431 = Concatenate Strings(w1259, w1248) -> (w1247:string)
                }
                n432 = Concatenate Strings(w1245) -> (w1246:string)
                n433 = String Length(string=w1246) -> (length=w1237:i32)
                n434 = Subtract(x=w1237, y=w1239) -> (x-y=w1238:i32)
                n435 = String Subset(string=w1246, length (rest)=w1238) -> (substring=w1241:string)  [unwired: 1 in]
                n436 = String Subset(string="====", length (rest)=w1239) -> (substring=w1242:string)  [unwired: 1 in]
                n437 = Concatenate Strings(w1241, w1242) -> (w1243:string)
              }
            }
          }
        }
      }
    }
    frame Error {
    }
  }
  "error out" <- w10
  "CypheredText out" <- w1
